vi "MC_10_19a.vi"() -> ()   [LabVIEW 2011]
uses:
  <vilib>/Utility/file.llb/Read From Spreadsheet File (string).vi
  <vilib>/Utility/inputDevices.llb/keyboardAcquire.vi
  <vilib>/Utility/file.llb/Write To Spreadsheet File (string).vi
  <vilib>/regexp/Match Regular Expression.xnode
panel:
  in  "Save Changes? 3":bool
  out "String":string
  in  "No Image":path=path "C:/Program Files/Mega Awesome/Image Not Found.png"
  in  "Save Changes? 2":bool
  in  "Project":path=path "C:/Program Files/Mega Awesome/DeviceData.opj"
  out "On/Off":dbl format="%#_3e"
  out "STS recorded":dbl
  out "Vt recorded":dbl
  out "Index 2":dbl
  out "Array 8":dbl[](array[numeric])
  out "Array 7":dbl[](array[numeric])
  in  "NumPts 2":dbl=5.0
  out "New S.T.S.":dbl
  out "S.T.S.":dbl
  in  "Slide 2":dbl(slide) step=1.0 scale=-1.0..82.0 scale format="%#_1p"
  in  "Previous Button 2":bool
  in  "Next Button 2":bool
  out "XY Graph 2":cluster{dbl[], dbl[]}[](graph)
  in  "Manual":bool
  out "New Vt":dbl
  out "Threshold V":dbl
  in  "Export":bool
  out "Image Name":string
  out "File":path
  out "Index":string
  out "Recorded Mobility":dbl format="%#_4e"
  in  "Remove Button":bool
  in  "Undo Button":bool
  out "Distances":dbl[](array[numeric])
  out "Total Width":dbl
  in  "Magnification":u16(ring) items=["5x", "10x", "20x", "50x", "80x"]
  out "Image Out":T1(plugin-control)
  in  "Folder":path
  out "Image Out 2":T1(plugin-control)
  out "ROI Descriptor out":T2 {"Contours"."Type" items=["No Selection", "Point", "Line", "Rectangle", "Oval", "Polygon", "Freehand Region", "Annulus", "Unused2", "Unused3", "Broken Line", "Freehand Line", "Rotated Rectangle"]}
  out "ROI Descriptor":T2 {"Contours"."Type" items=["No Selection", "Point", "Line", "Rectangle", "Oval", "Polygon", "Freehand Region", "Annulus", "Unused2", "Unused3", "Broken Line", "Freehand Line", "Rotated Rectangle"]}
  in  "Zoom":i16(slide)=-3 scale=-5.0..5.0
  out "Numeric 3":dbl
  in  "Blank Button":bool
  out "Array 6":dbl[][](array[numeric])
  out "Cluster":T3
  out "Array 5":dbl[](array[numeric])
  out "Array 4":dbl[](array[numeric])
  out "Array 3":dbl[](array[numeric])
  out "Numeric 2":dbl
  out "Numeric":dbl
  in  "Slide":dbl(slide) step=1.0 scale=-14.3..82.0 scale format="%#_1p"
  out "New Mobility":dbl format="%#_4e"
  out "Array 2":dbl[](array[numeric])
  out "Array":dbl[](array[numeric])
  in  "New Width":dbl
  in  "New Length":dbl
  in  "New Dielectric":dbl
  in  "Save Changes?":bool
  out "Index":dbl
  out "Data Name":string
  out "Folder":path
  in  "Down Button":bool
  in  "Up Button":bool
  in  "Previous Button":bool
  in  "Next Button":bool
  in  "Cancel Button":bool
  in  "NumPts":dbl=5.0
  out "XY Graph":cluster{dbl[], dbl[]}[](graph)
  out "Dielectric (d)":dbl
  out "Width":dbl
  out "Length":dbl
  out "Table Control 2":string[][](table)
  out "Table Control":string[][](table)
  in  "Row Start":dbl=20.0
  in  "File":path
  out "Mobility":dbl format="%#_4e"
  # "Data Location"
  # "Image Location"
  # "Recorded"
  # "Calculated"
  # "Re-Calculated"
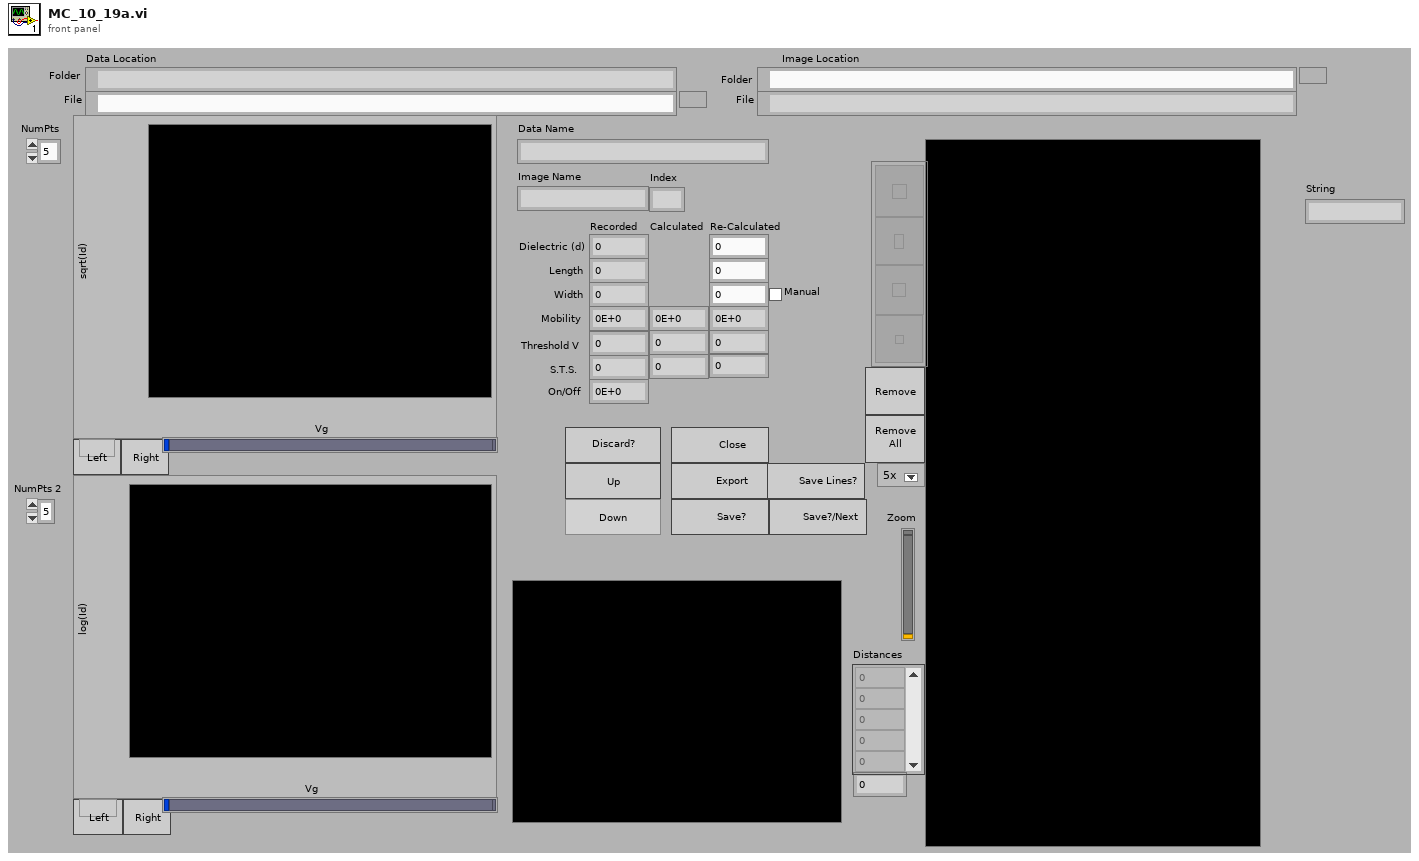
[diagram p1: front panel]
types:
  T1 = typedef "IMAQ Image.ctl" = refnum<image>
  T2 = typedef "ROI Descriptor" = cluster{"Global Rectangle":i32[], "Contours":cluster{"ID":enum32{"External", "Internal"}, "Type":u32, "Coordinates":i32[]}[]}
  T3 = cluster{"Numeric":dbl, "Numeric 2":dbl, "Numeric 3":dbl, "Numeric 4":dbl}
  T4 = cluster{"[0]":cluster{dbl[], dbl[]}, "[1]":cluster{dbl[], dbl[]}, "[2]":cluster{dbl[], dbl[]}, "[3]":cluster{dbl[], dbl[]}, "[4]":cluster{dbl[], dbl[]}, "[5]":cluster{dbl[], dbl[]}, "[6]":cluster{dbl[], dbl[]}, "[7]":cluster{dbl[], dbl[]}, "[8]":cluster{dbl[], dbl[]}}
  T5 = cluster{"Global Rectangle":i32[], "Contours":cluster{"Contour Type":u32, "ROI Type":u32, "Points":i32[]}[]}
  T6 = typedef "LVBoundsTypeDef.ctl" = cluster{"Width":u32, "Height":u32}
  T7 = cluster{"Contour Type":u32, "ROI Type":u32, "Points":i32[]}[]
  T8 = enum16{"0", "1", "2", "3", "4", "5", "6", "7", "8", "9", "A", "B", "C", "D", "E", "F", "G", "H", "I", "J", "K", "L", "M", "N", "O", "P", "Q", "R", "S", "T", "U", "V", "W", "X", "Y", "Z", "F1", "F2", "F3", "F4", "F5", "F6", "F7", "F8", "F9", "F10", "F11", "F12", "F13", "F14", "F15", "ADD", "BACK", "BACKSLASH", "CAPITAL", "COMMA", "DECIMAL", "DELETE", "DIVIDE", "DOWN", "END", "EQUALS", "ESCAPE", "GRAVE (`)", "HOME", "INSERT", "LBRACKET", "LCONTROL", "LEFT", "L ALT", "LSHIFT", "LWIN", "MINUS", "MULTIPLY", "NEXT", "NUMLOCK", "NUMPAD_0", "NUMPAD_1", "NUMPAD_2", "NUMPAD_3", "NUMPAD_4", "NUMPAD_5", "NUMPAD_6", "NUMPAD_7", "NUMPAD_8", "NUMPAD_9", "PAUSE", "PERIOD", "PRIOR (PG UP)", "RBRACKET", "RCONTROL", "RETURN", "RIGHT", "R ALT", "RSHIFT", "RWIN", "SCROLL", "SEMICOLON", "SLASH", "SPACE", "SUBTRACT", "TAB", "UP", "ENTER (num pad)", "' (quote)"}[]
  T9 = cluster{i32[], cluster{"Contour Type":u32, "ROI Type":u32, "Points":i32[]}[]}
  T10 = enum16{"0", "1", "2", "3", "4", "5", "6", "7", "8", "9", "A", "B", "C", "D", "E", "F", "G", "H", "I", "J", "K", "L", "M", "N", "O", "P", "Q", "R", "S", "T", "U", "V", "W", "X", "Y", "Z", "F1", "F2", "F3", "F4", "F5", "F6", "F7", "F8", "F9", "F10", "F11", "F12", "F13", "F14", "F15", "ADD", "BACK", "BACKSLASH", "CAPITAL", "COMMA", "DECIMAL", "DELETE", "DIVIDE", "DOWN", "END", "EQUALS", "ESCAPE", "GRAVE (`)", "HOME", "INSERT", "LBRACKET", "LCONTROL", "LEFT", "L ALT", "LSHIFT", "LWIN", "MINUS", "MULTIPLY", "NEXT", "NUMLOCK", "NUMPAD_0", "NUMPAD_1", "NUMPAD_2", "NUMPAD_3", "NUMPAD_4", "NUMPAD_5", "NUMPAD_6", "NUMPAD_7", "NUMPAD_8", "NUMPAD_9", "PAUSE", "PERIOD", "PRIOR (PG UP)", "RBRACKET", "RCONTROL", "RETURN", "RIGHT", "R ALT", "RSHIFT", "RWIN", "SCROLL", "SEMICOLON", "SLASH", "SPACE", "SUBTRACT", "TAB", "UP", "ENTER (num pad)", "' (quote)"}
  T11 = cluster{string, sgl, bool, bool, bool, bool, bool, bool, i32}
  T12 = cluster{i32, cluster{string, sgl, bool, bool, bool, bool, bool, bool, i32}, i32, i32}
  T13 = cluster{"Contour Type":u32, "ROI Type":u32, "Points":i32[]}
  T14 = cluster{"Points[0]":i32, "Points[1]":i32, "Points[2]":i32, "Points[3]":i32, "Points[4]":i32, "Points[5]":i32, "Points[6]":i32, "Points[7]":i32, "Points[8]":i32}
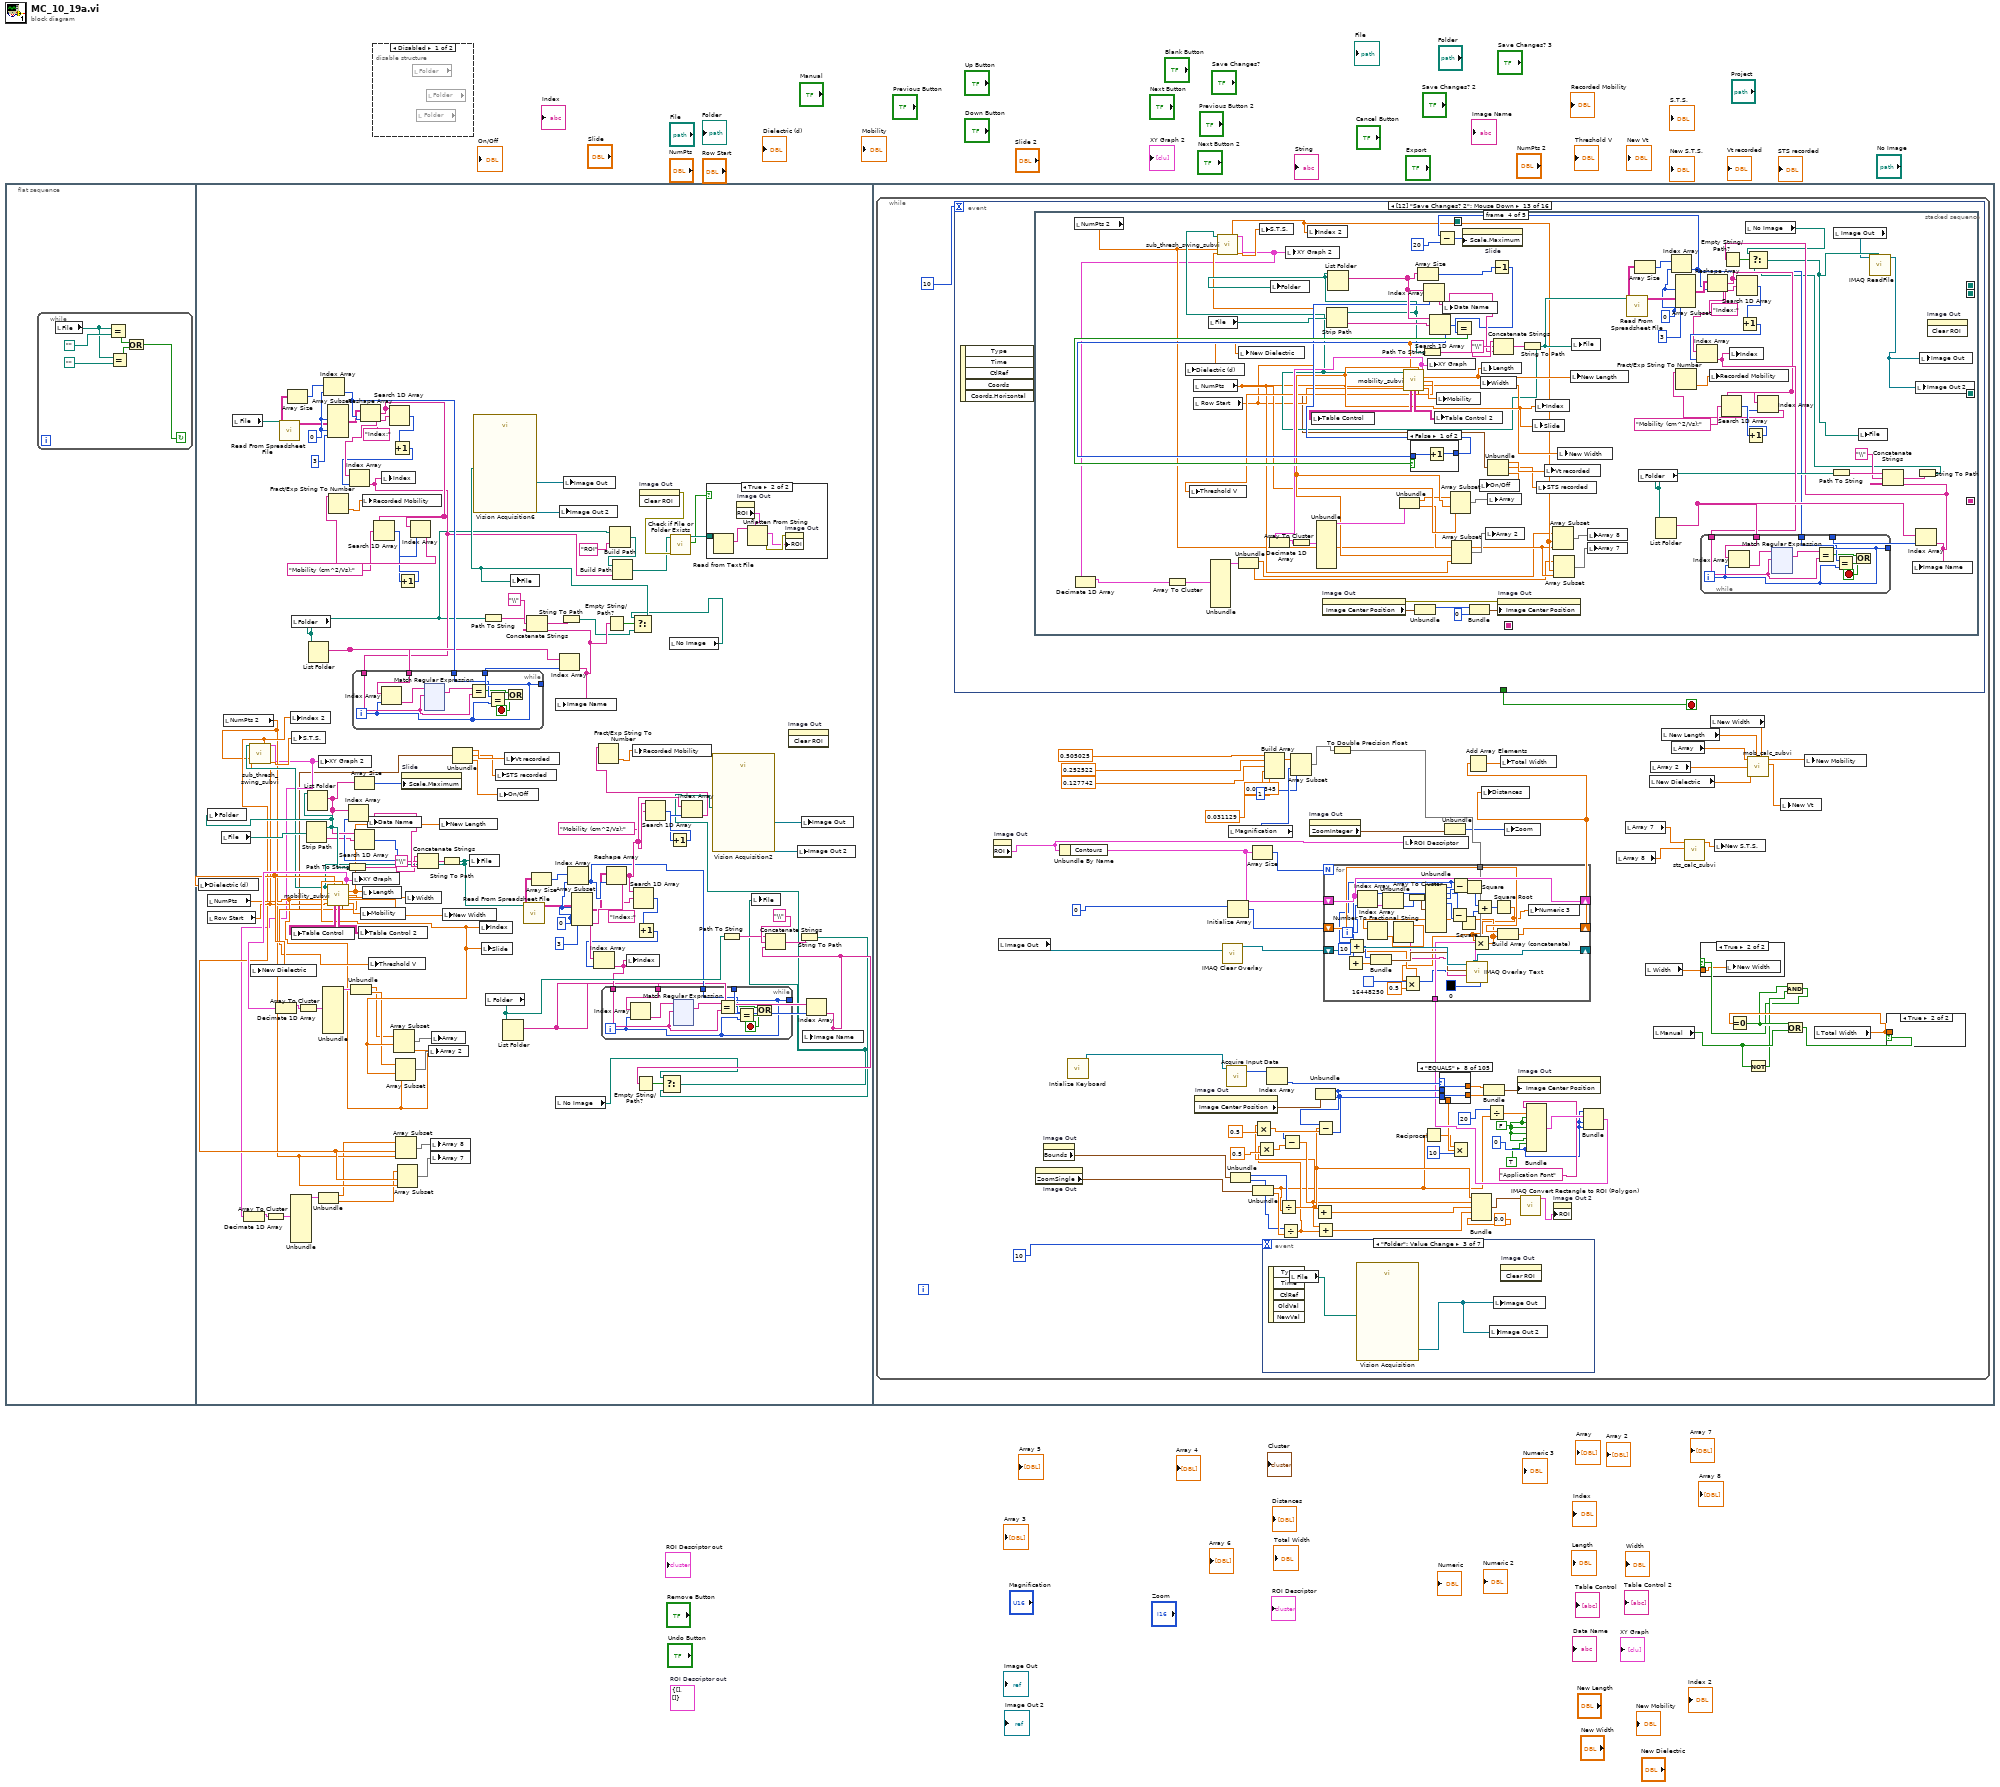
[diagram p0: block diagram]
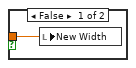
[diagram p4: hidden frame]
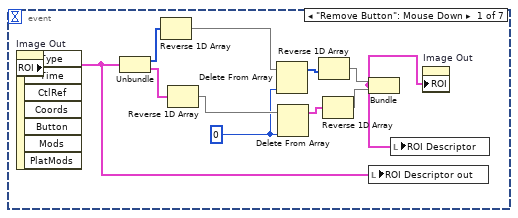
[diagram p5: hidden frame]
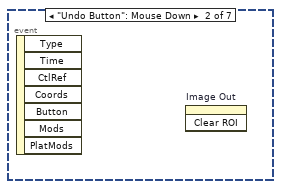
[diagram p6: hidden frame]
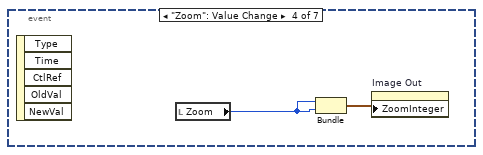
[diagram p7: hidden frame]
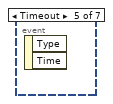
[diagram p8: hidden frame]
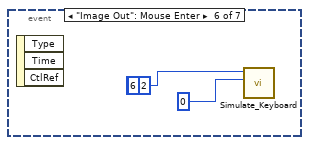
[diagram p9: hidden frame]
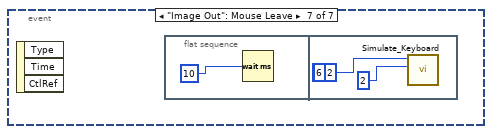
[diagram p10: hidden frame]
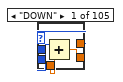
[diagram p11: hidden frame]
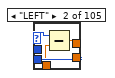
[diagram p12: hidden frame]
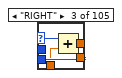
[diagram p13: hidden frame]
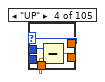
[diagram p14: hidden frame]
diagram:
  (unwired) T2 {"Global Rectangle"=[], "Contours"=[]}  # ROI Descriptor out
  n1 = flat-sequence {
    frame #0 {
      n2 = while {
        stop <- w1 continue-if-true
        n3 = local read "File"() -> (w3:path)
        n4 = Equal?(x=w3, y=path "") -> (x = y?=w5:bool)
        n5 = Equal?(x=w3, y=path "") -> (x = y?=w4:bool)
        n6 = Or(x=w5, y=w4) -> (x .or. y?=w1:bool)
      }
    }
    frame #1 {
      w67 = 0
      w97 = 0
      n7 = local read "NumPts"() -> (w42:dbl)
      n8 = local read "Row Start"() -> (w41:dbl)
      n9 = local read "File"() -> (w71:path)
      n10 = local read "NumPts 2"() -> (w36:dbl)
      n11 = local read "File"() -> (w92:path)
      n12 = call-poly <vilib>:"Read From Spreadsheet File.vi"("file path (dialog if empty)"=w92) -> ("all rows"=w95:string[][])  [unwired: 6 in, 4 out]
      n13 = Array Size(array=w95) -> (size(s)=w96:i32[])
      n14 = local read "Folder"() -> (w7:path)
      n15 = Strip Path(path=w71) -> (stripped path=w72:path, name=w53:string)
      n16 = local write "Folder"(w72) -> ()
      n17 = List Folder(path=w72) -> (filenames=w61:string[])  [unwired: 3 in, 3 out]
      n18 = List Folder(path=w7) -> (filenames=w101:string[])  [unwired: 3 in, 3 out]
      n19 = Index Array(array=w96, index=w97) -> (element=w103:i32)
      n20 = Array Subset(array=w95, index (row)=w97, index (col)=w97, length (col)=3) -> (w94:string[][])  [unwired: 1 in]
      n21 = Path To String(path=w72) -> (string=w52:string)
      n22 = Array Size(array=w61) -> (size(s)=w62:i32)
      n23 = Search 1D Array(1D array=w61, element=w53) -> (index of element=w60:i32)  [unwired: 1 in]
      n24 = Index Array(array=w61, index=w60) -> (element=w59:string)
      n25 = Reshape Array(w94, w103) -> (w113:string[])
      n26 = local write "Data Name"(w59) -> ()
      n27 = Search 1D Array(1D array=w113, element="Mobility (cm^2/Vs):") -> (index of element=w108:i32)  [unwired: 1 in]
      n28 = Search 1D Array(1D array=w113, element="Index:") -> (index of element=w100:i32)  [unwired: 1 in]
      n29 = Increment(x=w100) -> (x+1=w99:i32)
      n30 = Index Array(array=w113, index=w99) -> (element=w8:string)
      n31 = while {
        tunnel: w101 -> [w246]
        tunnel: w8 -> [w244]
        tunnel: [w243] -> _
        tunnel: [w243] -> w102
        tunnel: w103 -> [w242]
        i -> [w243]
        stop <- w239 stop-if-true
        n32 = Index Array(array=w246, index=w243) -> (element=w247:string)
        n33 = xnode "Match Regular Expression"("input string"=w247, "regular expression"=w244) -> ("whole match"=w245:string)  [unwired: 4 in, 4 out]
        n34 = Equal?(x=w245, y=w244) -> (x = y?=w241:bool)
        n35 = Equal?(x=w242, y=w243) -> (x = y?=w240:bool)
        n36 = Or(x=w241, y=w240) -> (x .or. y?=w239:bool)
      }
      n37 = local write "Index"(w8) -> ()
      n38 = Increment(x=w108) -> (x+1=w109:i32)
      n39 = property on="Slide" class="Slide (strict)"("Scale.Maximum"=w62) -> ()  [unwired: 2 in, 2 out]
      n40 = Index Array(array=w113, index=w109) -> (element=w111:string)
      n41 = Fract/Exp String To Number(string=w111) -> (number=w112:dbl)  [unwired: 3 in, 1 out]
      n42 = local write "Recorded Mobility"(w112) -> ()
      n43 = Concatenate Strings(w52, "\\", w59) -> (w54:string)
      n44 = String To Path(string=w54) -> (path=w43:path)
      n45 = call "sub_thresh_swing_subvi.vi"("Path"=w43, "NumPts"=w36, "Row Start"=w41) -> ("Index"=w37:dbl, "XY Graph"=w32:cluster{dbl[], dbl[]}[], "Sub Threshold Swing"=w44:dbl)  [unwired: 8 in, 2 out]
      n46 = Decimate 1D Array(w32) -> (w33:cluster{dbl[], dbl[]}[])  [unwired: 1 out]
      n47 = Array To Cluster(array=w33) -> (cluster=w35:T4)
      n48 = local write "Index 2"(w37) -> ()
      n49 = Unbundle(w35) -> ("[0]"=w34:cluster{dbl[], dbl[]})  [unwired: 8 out]
      n50 = local write "S.T.S."(w44) -> ()
      n51 = local write "XY Graph 2"(w32) -> ()
      n52 = Unbundle(w34) -> (w30:dbl[], w29:dbl[])
      n53 = call "mobility_subvi.vi"("Path"=w43, "NumPts"=w42, "Row Start"=w41) -> ("Dielectric (d)"=w48:dbl, "Index"=w49:dbl, "XY Graph"=w91:cluster{dbl[], dbl[]}[], "Length"=w47:dbl, "Vt"=w45:dbl, "Width"=w46:dbl, "Table Control"=w56:string[][], "Table Control 2"=w57:string[][], "Recorded"=w26:cluster{"Vt":dbl, "STS":dbl, "On/Off":dbl}, "Mobility"=w58:dbl)  [unwired: 3 in]
      n54 = local write "Dielectric (d)"(w48) -> ()
      n55 = local write "New Dielectric"(w48) -> ()
      n56 = Decimate 1D Array(w91) -> (w90:cluster{dbl[], dbl[]}[])  [unwired: 1 out]
      n57 = local write "Table Control"(w56) -> ()
      n58 = Array To Cluster(array=w90) -> (cluster=w88:T4)
      n59 = Unbundle(w88) -> ("[0]"=w89:cluster{dbl[], dbl[]})  [unwired: 8 out]
      n60 = Unbundle(w89) -> (w31:dbl[], w38:dbl[])
      n61 = local write "XY Graph"(w91) -> ()
      n62 = local write "Table Control 2"(w57) -> ()
      n63 = local write "Mobility"(w58) -> ()
      n64 = local write "Length"(w47) -> ()
      n65 = local write "Threshold V"(w45) -> ()
      n66 = Array Subset(array=w31, index=w49, length=w42) -> (w50:dbl[])
      n67 = Array Subset(array=w38, index=w49, length=w42) -> (w51:dbl[])
      n68 = Array Subset(array=w30, index=w37, length=w36) -> (w40:dbl[])
      n69 = Array Subset(array=w29, index=w37, length=w36) -> (w39:dbl[])
      n70 = local write "Width"(w46) -> ()
      n71 = local write "Array 2"(w51) -> ()
      n72 = local write "Array 8"(w40) -> ()
      n73 = local write "Array 7"(w39) -> ()
      n74 = local write "Array"(w50) -> ()
      n75 = local write "New Length"(w47) -> ()
      n76 = local write "New Width"(w46) -> ()
      n77 = Unbundle(w26) -> ("Vt"=w28:dbl, "STS"=w27:dbl, "On/Off"=w25:dbl)
      n78 = local write "File"(w43) -> ()
      n79 = local write "Index"(w49) -> ()
      n80 = local write "Slide"(w49) -> ()
      n81 = Path To String(path=w7) -> (string=w105:string)
      n82 = local read "Folder"() -> (w78:path)
      n83 = local write "STS recorded"(w27) -> ()
      n84 = local write "On/Off"(w25) -> ()
      n85 = List Folder(path=w78) -> (filenames=w74:string[])  [unwired: 3 in, 3 out]
      n86 = local write "Vt recorded"(w28) -> ()
      n87 = call-poly <vilib>:"Read From Spreadsheet File.vi"("file path (dialog if empty)"=w43) -> ("all rows"=w65:string[][])  [unwired: 6 in, 4 out]
      n88 = Array Size(array=w65) -> (size(s)=w66:i32[])
      n89 = local read "No Image"() -> (w16:path)
      n90 = Index Array(array=w101, index=w102) -> (element=w24:string)
      n91 = Concatenate Strings(w105, "\\", w24) -> (w106:string)
      n92 = local write "Image Name"(w24) -> ()
      n93 = String To Path(string=w106) -> (path=w22:path)
      n94 = Index Array(array=w66, index=w67) -> (element=w77:i32)
      n95 = Array Subset(array=w65, index (row)=w67, index (col)=w67, length (col)=3) -> (w64:string[][])  [unwired: 1 in]
      n96 = Empty String/Path?(string/path=w24) -> (empty?=w23:bool)
      n97 = Reshape Array(w64, w77) -> (w87:string[])
      n98 = Build Path(base path=w7, name or relative path="ROI") -> (appended path=w10:path)
      n99 = Build Path(base path=w10, name or relative path=w8) -> (appended path=w9:path)
      n100 = Search 1D Array(1D array=w87, element="Index:") -> (index of element=w70:i32)  [unwired: 1 in]
      n101 = Increment(x=w70) -> (x+1=w69:i32)
      n102 = Index Array(array=w87, index=w69) -> (element=w75:string)
      n103 = while {
        tunnel: w74 -> [w126]
        tunnel: w75 -> [w124]
        tunnel: [w123] -> _
        tunnel: [w123] -> w76
        tunnel: w77 -> [w122]
        i -> [w123]
        stop <- w119 stop-if-true
        n104 = Index Array(array=w126, index=w123) -> (element=w127:string)
        n105 = xnode "Match Regular Expression"("input string"=w127, "regular expression"=w124) -> ("whole match"=w125:string)  [unwired: 4 in, 4 out]
        n106 = Equal?(x=w125, y=w124) -> (x = y?=w121:bool)
        n107 = Equal?(x=w122, y=w123) -> (x = y?=w120:bool)
        n108 = Or(x=w121, y=w120) -> (x .or. y?=w119:bool)
      }
      n109 = local write "Index"(w75) -> ()
      n110 = invoke on="Image Out" class="ImageControl" method="Clear ROI"() -> (error out=w14:errorcluster)  [unwired: 3 in, 2 out]
      n111 = Search 1D Array(1D array=w87, element="Mobility (cm^2/Vs):") -> (index of element=w82:i32)  [unwired: 1 in]
      n112 = local read "No Image"() -> (w15:path)
      n113 = Select(t=w15, s=w23, f=w22) -> (s? t:f=w21:path)
      n114 = call "Vision Acquisition6"("Image Path"=w21) -> ("Image Out"=w104:T1)  [unwired: 25 in, 1 out]
      n115 = local write "File"(w21) -> ()
      n116 = local write "Image Out 2"(w104) -> ()
      n117 = local write "Image Out"(w104) -> ()
      n118 = Increment(x=w82) -> (x+1=w83:i32)
      n119 = call <vilib>:"Check if File or Folder Exists.vi"("error in (no error)"=w14, "path"=w9) -> ("file or folder exists?"=w12:bool, "dup path"=w13:path)  [unwired: 7 in, 1 out]
      n120 = Index Array(array=w87, index=w83) -> (element=w85:string)
      n121 = Fract/Exp String To Number(string=w85) -> (number=w86:dbl)  [unwired: 3 in, 1 out]
      n122 = local write "Recorded Mobility"(w86) -> ()
      n123 = case shown="True" w12 {
        tunnel: w13 -> [_ w114]
        frame False {
        }
        frame True {
          n124 = Read from Text File(file (use dialog)=w114) -> (text=w118:string)  [unwired: 3 in, 3 out]
          n125 = property on="Image Out" class="ImageControl"() -> ("ROI"=w115:T5)  [unwired: 2 in, 2 out]
          n126 = Unflatten From String(type=w115, binary string=w118) -> (value=w116:T5, error out=w117:errorcluster)  [unwired: 3 in, 1 out]
          n127 = property on="Image Out" class="ImageControl"(error in=w117, "ROI"=w116) -> ()  [unwired: 1 in, 2 out]
        }
      }
      n128 = Path To String(path=w78) -> (string=w79:string)
      n129 = invoke on="Image Out" class="ImageControl" method="Clear ROI"() -> ()  [unwired: 3 in, 3 out]
      n130 = Index Array(array=w74, index=w76) -> (element=w19:string)
      n131 = Empty String/Path?(string/path=w19) -> (empty?=w20:bool)
      n132 = Concatenate Strings(w79, "\\", w19) -> (w80:string)
      n133 = String To Path(string=w80) -> (path=w18:path)
      n134 = Select(t=w16, s=w20, f=w18) -> (s? t:f=w17:path)
      n135 = call "Vision Acquisition2"("Image Path"=w17) -> ("Image Out"=w73:T1)  [unwired: 25 in, 1 out]
      n136 = local write "File"(w17) -> ()
      n137 = local write "Image Out 2"(w73) -> ()
      n138 = local write "Image Out"(w73) -> ()
      n139 = local write "Image Name"(w19) -> ()
    }
    frame #2 {
      n140 = while {
        stop <- w438 stop-if-true
        w388 = FALSE
        w386 = 0
        n141 = event shown="[12] \"Save Changes? 2\": Mouse Down" {
          selector: _ -> [_ _ _ _ _ _ _ _ _ _ _ _ _ _ _ _]
          dyn-events: _ -> [_ _ _ _ _ _ _ _ _ _ _ _ _ _ _ _]
          timeout: 10 -> [_ _ _ _ _ _ _ _ _ _ _ _ _ _ _ _]
          tunnel: [_ _ _ _ _ _ _ _ _ _ _ _ _ TRUE _ TRUE] -> w438
          event Timeout {
            n142 = event-data() -> ()  [unwired: 1 in, 2 out]
          }
          event "Down Button": Mouse Down {
            w781 = 0
            n143 = event-data() -> ()  [unwired: 1 in, 7 out]
            n144 = local read "NumPts 2"() -> (w742:dbl)
            n145 = local read "NumPts"() -> (w749:dbl)
            n146 = local read "Row Start"() -> (w748:dbl)
            n147 = local read "File"() -> (w786:path)
            n148 = property on="Image Out" class="ImageControl"() -> (error out=w711:errorcluster, "Image Center Position"=w715:cluster{"X":u32, "Y":u32})  [unwired: 2 in, 1 out]
            n149 = Unbundle(w715) -> ("X"=w713:u32)  [unwired: 1 out]
            n150 = Strip Path(path=w786) -> (stripped path=w777:path, name=w799:string)
            n151 = local write "Folder"(w777) -> ()
            n152 = List Folder(path=w777) -> (filenames=w792:string[], error out=w720:errorcluster)  [unwired: 3 in, 2 out]
            n153 = Array Size(array=w792) -> (size(s)=w787:i32)
            n154 = Bundle("X"=w713, 0) -> (w714:cluster{"X":u32, i32})  [unwired: 1 in]
            n155 = Path To String(path=w777) -> (string=w800:string)
            n156 = Search 1D Array(1D array=w792, element=w799) -> (index of element=w789:i32)  [unwired: 1 in]
            n157 = property on="Image Out" class="ImageControl"(error in=w711, "Image Center Position"=w714) -> ()  [unwired: 1 in, 2 out]
            n158 = Decrement(x=w787) -> (x-1=w790:i32)
            n159 = Equal?(x=w789, y=w790) -> (x = y?=w791:bool)
            n160 = case shown="False" w791 {
              tunnel: w789 -> [w927 _]
              tunnel: [w926 0] -> w788
              frame False {
                n161 = Increment(x=w927) -> (x+1=w926:i32)
              }
              frame True {
              }
            }
            n162 = Index Array(array=w792, index=w788) -> (element=w793:string)
            n163 = local write "Data Name"(w793) -> ()
            n164 = Concatenate Strings(w800, "\\", w793) -> (w798:string)
            n165 = String To Path(string=w798) -> (path=w750:path)
            n166 = call "sub_thresh_swing_subvi.vi"("Path"=w750, "NumPts"=w742, "Row Start"=w748) -> ("Index"=w743:dbl, "XY Graph"=w738:cluster{dbl[], dbl[]}[], "Sub Threshold Swing"=w751:dbl)  [unwired: 8 in, 2 out]
            n167 = Decimate 1D Array(w738) -> (w741:cluster{dbl[], dbl[]}[])  [unwired: 1 out]
            n168 = Array To Cluster(array=w741) -> (cluster=w739:T4)
            n169 = Unbundle(w739) -> ("[0]"=w740:cluster{dbl[], dbl[]})  [unwired: 8 out]
            n170 = Unbundle(w740) -> (w737:dbl[], w736:dbl[])
            n171 = local write "S.T.S."(w751) -> ()
            n172 = local write "XY Graph 2"(w738) -> ()
            n173 = local write "Index 2"(w743) -> ()
            n174 = call "mobility_subvi.vi"("Path"=w750, "NumPts"=w749, "Row Start"=w748) -> ("Dielectric (d)"=w753:dbl, "Index"=w758:dbl, "XY Graph"=w761:cluster{dbl[], dbl[]}[], "Length"=w752:dbl, "Vt"=w754:dbl, "Width"=w726:dbl, "Table Control"=w796:string[][], "Table Control 2"=w795:string[][], "Recorded"=w735:cluster{"Vt":dbl, "STS":dbl, "On/Off":dbl}, "Mobility"=w794:dbl)  [unwired: 3 in]
            n175 = local write "Dielectric (d)"(w753) -> ()
            n176 = local write "Threshold V"(w754) -> ()
            n177 = local write "New Dielectric"(w753) -> ()
            n178 = Decimate 1D Array(w761) -> (w762:cluster{dbl[], dbl[]}[])  [unwired: 1 out]
            n179 = Array To Cluster(array=w762) -> (cluster=w764:T4)
            n180 = local write "Table Control"(w796) -> ()
            n181 = Unbundle(w764) -> ("[0]"=w763:cluster{dbl[], dbl[]})  [unwired: 8 out]
            n182 = Unbundle(w763) -> (w745:dbl[], w744:dbl[])
            n183 = local write "XY Graph"(w761) -> ()
            n184 = local write "Table Control 2"(w795) -> ()
            n185 = local write "Mobility"(w794) -> ()
            n186 = Array Subset(array=w745, index=w758, length=w749) -> (w760:dbl[])
            n187 = Array Subset(array=w744, index=w758, length=w749) -> (w759:dbl[])
            n188 = local write "Width"(w726) -> ()
            n189 = local write "Length"(w752) -> ()
            n190 = local write "Array 2"(w759) -> ()
            n191 = Unbundle(w735) -> ("Vt"=w734:dbl, "STS"=w733:dbl, "On/Off"=w732:dbl)
            n192 = local write "On/Off"(w732) -> ()
            n193 = local write "Array"(w760) -> ()
            n194 = local write "Slide"(w758) -> ()
            n195 = local write "Index"(w758) -> ()
            n196 = local write "STS recorded"(w733) -> ()
            n197 = local write "Vt recorded"(w734) -> ()
            n198 = Array Subset(array=w737, index=w743, length=w742) -> (w747:dbl[])
            n199 = Array Subset(array=w736, index=w743, length=w742) -> (w746:dbl[])
            n200 = local write "New Width"(w726) -> ()
            n201 = local write "New Length"(w752) -> ()
            n202 = local write "File"(w750) -> ()
            n203 = local write "Array 8"(w747) -> ()
            n204 = local write "Array 7"(w746) -> ()
            n205 = call-poly <vilib>:"Read From Spreadsheet File.vi"("file path (dialog if empty)"=w750) -> ("all rows"=w783:string[][])  [unwired: 6 in, 4 out]
            n206 = Array Size(array=w783) -> (size(s)=w782:i32[])
            n207 = local read "Folder"() -> (w717:path)
            n208 = List Folder(path=w717, error in=w720) -> (filenames=w776:string[], error out=w721:errorcluster)  [unwired: 2 in, 2 out]
            n209 = Index Array(array=w782, index=w781) -> (element=w756:i32)
            n210 = Subtract(x=w756, y=20) -> (x-y=w755:i32)
            n211 = property on="Slide" class="Slide (strict)"("Scale.Maximum"=w755) -> ()  [unwired: 2 in, 2 out]
            n212 = Array Subset(array=w783, index (row)=w781, index (col)=w781, length (col)=3) -> (w784:string[][])  [unwired: 1 in]
            n213 = Reshape Array(w784, w756) -> (w765:string[])
            n214 = local read "No Image"() -> (w727:path)
            n215 = Search 1D Array(1D array=w765, element="Mobility (cm^2/Vs):") -> (index of element=w770:i32)  [unwired: 1 in]
            n216 = Search 1D Array(1D array=w765, element="Index:") -> (index of element=w778:i32)  [unwired: 1 in]
            n217 = Increment(x=w778) -> (x+1=w779:i32)
            n218 = Index Array(array=w765, index=w779) -> (element=w719:string)
            n219 = while {
              tunnel: w776 -> [w813]
              tunnel: w719 -> [w811]
              tunnel: [w810] -> _
              tunnel: [w810] -> w775
              tunnel: w756 -> [w809]
              i -> [w810]
              stop <- w806 stop-if-true
              n220 = Index Array(array=w813, index=w810) -> (element=w814:string)
              n221 = xnode "Match Regular Expression"("input string"=w814, "regular expression"=w811) -> ("whole match"=w812:string)  [unwired: 4 in, 4 out]
              n222 = Equal?(x=w812, y=w811) -> (x = y?=w808:bool)
              n223 = Equal?(x=w809, y=w810) -> (x = y?=w807:bool)
              n224 = Or(x=w808, y=w807) -> (x .or. y?=w806:bool)
            }
            n225 = local write "Index"(w719) -> ()
            n226 = Increment(x=w770) -> (x+1=w769:i32)
            n227 = Build Path(base path=w717, name or relative path="ROI") -> (appended path=w716:path)
            n228 = Index Array(array=w765, index=w769) -> (element=w767:string)
            n229 = Fract/Exp String To Number(string=w767) -> (number=w766:dbl)  [unwired: 3 in, 1 out]
            n230 = local write "Recorded Mobility"(w766) -> ()
            n231 = Build Path(base path=w716, name or relative path=w719) -> (appended path=w725:path)
            n232 = Path To String(path=w717) -> (string=w773:string)
            n233 = invoke on="Image Out" class="ImageControl" method="Clear ROI"(error in=w721) -> (error out=w724:errorcluster)  [unwired: 2 in, 2 out]
            n234 = call <vilib>:"Check if File or Folder Exists.vi"("error in (no error)"=w724, "path"=w725) -> ("file or folder exists?"=w722:bool, "dup path"=w723:path)  [unwired: 7 in, 1 out]
            n235 = Index Array(array=w776, index=w775) -> (element=w730:string)
            n236 = Empty String/Path?(string/path=w730) -> (empty?=w731:bool)
            n237 = Concatenate Strings(w773, "\\", w730) -> (w772:string)
            n238 = local write "Image Name"(w730) -> ()
            n239 = String To Path(string=w772) -> (path=w729:path)
            n240 = Select(t=w727, s=w731, f=w729) -> (s? t:f=w728:path)
            n241 = call "Vision Acquisition4"("Image Path"=w728) -> ("Image Out"=w774:T1)  [unwired: 25 in, 1 out]
            n242 = local write "File"(w728) -> ()
            n243 = local write "Image Out 2"(w774) -> ()
            n244 = case shown="True" w722 {
              tunnel: w723 -> [_ w801]
              frame False {
              }
              frame True {
                n245 = Read from Text File(file (use dialog)=w801) -> (text=w805:string)  [unwired: 3 in, 3 out]
                n246 = property on="Image Out" class="ImageControl"() -> ("ROI"=w802:T5)  [unwired: 2 in, 2 out]
                n247 = Unflatten From String(type=w802, binary string=w805) -> (value=w803:T5, error out=w804:errorcluster)  [unwired: 3 in, 1 out]
                n248 = property on="Image Out" class="ImageControl"(error in=w804, "ROI"=w803) -> ()  [unwired: 1 in, 2 out]
              }
            }
            n249 = local write "Image Out"(w774) -> ()
            n250 = invoke on="Image Out" class="ImageControl" method="Clear ROI"() -> ()  [unwired: 3 in, 3 out]
          }
          event "File": Value Change {
            w1000 = 0
            n251 = event-data() -> ()  [unwired: 1 in, 5 out]
            n252 = local read "NumPts"() -> (w968:dbl)
            n253 = local read "Row Start"() -> (w967:dbl)
            n254 = local read "File"() -> (w996:path)
            n255 = local read "NumPts 2"() -> (w961:dbl)
            n256 = property on="Image Out" class="ImageControl"() -> (error out=w929:errorcluster, "Image Center Position"=w933:cluster{"X":u32, "Y":u32})  [unwired: 2 in, 1 out]
            n257 = Strip Path(path=w996) -> (stripped path=w995:path, name=w1013:string)
            n258 = local write "Folder"(w995) -> ()
            n259 = List Folder(path=w995) -> (filenames=w1005:string[], error out=w939:errorcluster)  [unwired: 3 in, 2 out]
            n260 = Unbundle(w933) -> ("X"=w931:u32)  [unwired: 1 out]
            n261 = Path To String(path=w995) -> (string=w1014:string)
            n262 = Search 1D Array(1D array=w1005, element=w1013) -> (index of element=w1006:i32)  [unwired: 1 in]
            n263 = Index Array(array=w1005, index=w1006) -> (element=w1007:string)
            n264 = Bundle("X"=w931, 0) -> (w932:cluster{"X":u32, i32})  [unwired: 1 in]
            n265 = local write "Data Name"(w1007) -> ()
            n266 = property on="Image Out" class="ImageControl"(error in=w929, "Image Center Position"=w932) -> ()  [unwired: 1 in, 2 out]
            n267 = Concatenate Strings(w1014, "\\", w1007) -> (w1012:string)
            n268 = String To Path(string=w1012) -> (path=w969:path)
            n269 = call "sub_thresh_swing_subvi.vi"("Path"=w969, "NumPts"=w961, "Row Start"=w967) -> ("Index"=w962:dbl, "XY Graph"=w957:cluster{dbl[], dbl[]}[], "Sub Threshold Swing"=w966:dbl)  [unwired: 8 in, 2 out]
            n270 = Decimate 1D Array(w957) -> (w960:cluster{dbl[], dbl[]}[])  [unwired: 1 out]
            n271 = Array To Cluster(array=w960) -> (cluster=w958:T4)
            n272 = Unbundle(w958) -> ("[0]"=w959:cluster{dbl[], dbl[]})  [unwired: 8 out]
            n273 = Unbundle(w959) -> (w955:dbl[], w954:dbl[])
            n274 = local write "Index 2"(w962) -> ()
            n275 = call "mobility_subvi.vi"("Path"=w969, "NumPts"=w968, "Row Start"=w967) -> ("Dielectric (d)"=w971:dbl, "Index"=w976:dbl, "XY Graph"=w979:cluster{dbl[], dbl[]}[], "Length"=w970:dbl, "Vt"=w972:dbl, "Width"=w944:dbl, "Table Control"=w1010:string[][], "Table Control 2"=w1009:string[][], "Recorded"=w951:cluster{"Vt":dbl, "STS":dbl, "On/Off":dbl}, "Mobility"=w1008:dbl)  [unwired: 3 in]
            n276 = local write "Dielectric (d)"(w971) -> ()
            n277 = local write "New Dielectric"(w971) -> ()
            n278 = Decimate 1D Array(w979) -> (w980:cluster{dbl[], dbl[]}[])  [unwired: 1 out]
            n279 = local write "Table Control"(w1010) -> ()
            n280 = Array To Cluster(array=w980) -> (cluster=w982:T4)
            n281 = Unbundle(w982) -> ("[0]"=w981:cluster{dbl[], dbl[]})  [unwired: 8 out]
            n282 = local write "Threshold V"(w972) -> ()
            n283 = local write "S.T.S."(w966) -> ()
            n284 = Unbundle(w981) -> (w956:dbl[], w963:dbl[])
            n285 = local write "XY Graph"(w979) -> ()
            n286 = local write "Table Control 2"(w1009) -> ()
            n287 = local write "Mobility"(w1008) -> ()
            n288 = local write "Length"(w970) -> ()
            n289 = local write "XY Graph 2"(w957) -> ()
            n290 = Unbundle(w951) -> ("Vt"=w953:dbl, "STS"=w952:dbl, "On/Off"=w950:dbl)
            n291 = local write "On/Off"(w950) -> ()
            n292 = Array Subset(array=w955, index=w962, length=w961) -> (w965:dbl[])
            n293 = Array Subset(array=w954, index=w962, length=w961) -> (w964:dbl[])
            n294 = local write "Width"(w944) -> ()
            n295 = Array Subset(array=w956, index=w976, length=w968) -> (w978:dbl[])
            n296 = Array Subset(array=w963, index=w976, length=w968) -> (w977:dbl[])
            n297 = local write "Array 8"(w965) -> ()
            n298 = local write "Array 7"(w964) -> ()
            n299 = local write "STS recorded"(w952) -> ()
            n300 = local write "Vt recorded"(w953) -> ()
            n301 = local write "New Length"(w970) -> ()
            n302 = local write "New Width"(w944) -> ()
            n303 = local write "Array 2"(w977) -> ()
            n304 = local write "Array"(w978) -> ()
            n305 = local write "File"(w969) -> ()
            n306 = local write "Index"(w976) -> ()
            n307 = local write "Slide"(w976) -> ()
            n308 = local read "Folder"() -> (w935:path)
            n309 = List Folder(path=w935, error in=w939) -> (filenames=w993:string[], error out=w938:errorcluster)  [unwired: 2 in, 2 out]
            n310 = call-poly <vilib>:"Read From Spreadsheet File.vi"("file path (dialog if empty)"=w969) -> ("all rows"=w1002:string[][])  [unwired: 6 in, 4 out]
            n311 = Array Size(array=w1002) -> (size(s)=w1001:i32[])
            n312 = Index Array(array=w1001, index=w1000) -> (element=w975:i32)
            n313 = Subtract(x=w975, y=20) -> (x-y=w973:i32)
            n314 = property on="Slide" class="Slide (strict)"("Scale.Maximum"=w973) -> ()  [unwired: 2 in, 2 out]
            n315 = Array Subset(array=w1002, index (row)=w1000, index (col)=w1000, length (col)=3) -> (w1003:string[][])  [unwired: 1 in]
            n316 = Reshape Array(w1003, w975) -> (w983:string[])
            n317 = Search 1D Array(1D array=w983, element="Index:") -> (index of element=w997:i32)  [unwired: 1 in]
            n318 = Increment(x=w997) -> (x+1=w998:i32)
            n319 = Index Array(array=w983, index=w998) -> (element=w937:string)
            n320 = while {
              tunnel: w993 -> [w1027]
              tunnel: w937 -> [w1025]
              tunnel: [w1024] -> _
              tunnel: [w1024] -> w992
              tunnel: w975 -> [w1023]
              i -> [w1024]
              stop <- w1020 stop-if-true
              n321 = Index Array(array=w1027, index=w1024) -> (element=w1028:string)
              n322 = xnode "Match Regular Expression"("input string"=w1028, "regular expression"=w1025) -> ("whole match"=w1026:string)  [unwired: 4 in, 4 out]
              n323 = Equal?(x=w1026, y=w1025) -> (x = y?=w1022:bool)
              n324 = Equal?(x=w1023, y=w1024) -> (x = y?=w1021:bool)
              n325 = Or(x=w1022, y=w1021) -> (x .or. y?=w1020:bool)
            }
            n326 = local write "Index"(w937) -> ()
            n327 = Search 1D Array(1D array=w983, element="Mobility (cm^2/Vs):") -> (index of element=w988:i32)  [unwired: 1 in]
            n328 = Increment(x=w988) -> (x+1=w987:i32)
            n329 = Index Array(array=w983, index=w987) -> (element=w985:string)
            n330 = Fract/Exp String To Number(string=w985) -> (number=w984:dbl)  [unwired: 3 in, 1 out]
            n331 = local write "Recorded Mobility"(w984) -> ()
            n332 = Build Path(base path=w935, name or relative path="ROI") -> (appended path=w934:path)
            n333 = Path To String(path=w935) -> (string=w991:string)
            n334 = local read "No Image"() -> (w945:path)
            n335 = Build Path(base path=w934, name or relative path=w937) -> (appended path=w943:path)
            n336 = invoke on="Image Out" class="ImageControl" method="Clear ROI"(error in=w938) -> (error out=w942:errorcluster)  [unwired: 2 in, 2 out]
            n337 = Index Array(array=w993, index=w992) -> (element=w948:string)
            n338 = Empty String/Path?(string/path=w948) -> (empty?=w949:bool)
            n339 = Concatenate Strings(w991, "\\", w948) -> (w990:string)
            n340 = String To Path(string=w990) -> (path=w947:path)
            n341 = Select(t=w945, s=w949, f=w947) -> (s? t:f=w946:path)
            n342 = call "Vision Acquisition3"("Image Path"=w946) -> ("Image Out"=w994:T1)  [unwired: 25 in, 1 out]
            n343 = local write "File"(w946) -> ()
            n344 = local write "Image Out 2"(w994) -> ()
            n345 = local write "Image Out"(w994) -> ()
            n346 = local write "Image Name"(w948) -> ()
            n347 = call <vilib>:"Check if File or Folder Exists.vi"("error in (no error)"=w942, "path"=w943) -> ("file or folder exists?"=w940:bool, "dup path"=w941:path)  [unwired: 7 in, 1 out]
            n348 = invoke on="Image Out" class="ImageControl" method="Clear ROI"() -> ()  [unwired: 3 in, 3 out]
            n349 = case shown="True" w940 {
              tunnel: w941 -> [_ w1015]
              frame False {
              }
              frame True {
                n350 = Read from Text File(file (use dialog)=w1015) -> (text=w1019:string)  [unwired: 3 in, 3 out]
                n351 = property on="Image Out" class="ImageControl"() -> ("ROI"=w1016:T5)  [unwired: 2 in, 2 out]
                n352 = Unflatten From String(type=w1016, binary string=w1019) -> (value=w1017:T5, error out=w1018:errorcluster)  [unwired: 3 in, 1 out]
                n353 = property on="Image Out" class="ImageControl"(error in=w1018, "ROI"=w1017) -> ()  [unwired: 1 in, 2 out]
              }
            }
          }
          event "Up Button": Mouse Down {
            w1211 = 0
            n354 = event-data() -> ()  [unwired: 1 in, 5 out]
            n355 = local read "NumPts"() -> (w1182:dbl)
            n356 = local read "Row Start"() -> (w1181:dbl)
            n357 = local read "NumPts 2"() -> (w1176:dbl)
            n358 = local read "File"() -> (w1207:path)
            n359 = property on="Image Out" class="ImageControl"() -> (error out=w1140:errorcluster, "Image Center Position"=w1144:cluster{"X":u32, "Y":u32})  [unwired: 2 in, 1 out]
            n360 = Strip Path(path=w1207) -> (stripped path=w1206:path, name=w1227:string)
            n361 = local write "Folder"(w1206) -> ()
            n362 = List Folder(path=w1206) -> (filenames=w1217:string[], error out=w1150:errorcluster)  [unwired: 3 in, 2 out]
            n363 = Path To String(path=w1206) -> (string=w1228:string)
            n364 = Search 1D Array(1D array=w1217, element=w1227) -> (index of element=w1219:i32)  [unwired: 1 in]
            n365 = Equal To 0?(x=w1219) -> (x = 0?=w1220:bool)
            n366 = Unbundle(w1144) -> ("X"=w1142:u32)  [unwired: 1 out]
            n367 = Bundle("X"=w1142, 0) -> (w1143:cluster{"X":u32, i32})  [unwired: 1 in]
            n368 = property on="Image Out" class="ImageControl"(error in=w1140, "Image Center Position"=w1143) -> ()  [unwired: 1 in, 2 out]
            n369 = Array Size(array=w1217) -> (size(s)=w1216:i32)
            n370 = case shown="True" w1220 {
              tunnel: w1219 -> [w1355 _]
              tunnel: [w1354 w1356] -> w1218
              tunnel: w1216 -> [_ w1357]
              frame False {
                n371 = Decrement(x=w1355) -> (x-1=w1354:i32)
              }
              frame True {
                n372 = Decrement(x=w1357) -> (x-1=w1356:i32)
              }
            }
            n373 = Index Array(array=w1217, index=w1218) -> (element=w1221:string)
            n374 = local write "Data Name"(w1221) -> ()
            n375 = Concatenate Strings(w1228, "\\", w1221) -> (w1226:string)
            n376 = String To Path(string=w1226) -> (path=w1183:path)
            n377 = call "sub_thresh_swing_subvi.vi"("Path"=w1183, "NumPts"=w1176, "Row Start"=w1181) -> ("Index"=w1175:dbl, "XY Graph"=w1171:cluster{dbl[], dbl[]}[], "Sub Threshold Swing"=w1184:dbl)  [unwired: 8 in, 2 out]
            n378 = Decimate 1D Array(w1171) -> (w1174:cluster{dbl[], dbl[]}[])  [unwired: 1 out]
            n379 = Array To Cluster(array=w1174) -> (cluster=w1172:T4)
            n380 = Unbundle(w1172) -> ("[0]"=w1173:cluster{dbl[], dbl[]})  [unwired: 8 out]
            n381 = Unbundle(w1173) -> (w1170:dbl[], w1169:dbl[])
            n382 = Array Subset(array=w1170, index=w1175, length=w1176) -> (w1178:dbl[])
            n383 = Array Subset(array=w1169, index=w1175, length=w1176) -> (w1177:dbl[])
            n384 = local write "S.T.S."(w1184) -> ()
            n385 = local write "Array 8"(w1178) -> ()
            n386 = local write "Array 7"(w1177) -> ()
            n387 = call "mobility_subvi.vi"("Path"=w1183, "NumPts"=w1182, "Row Start"=w1181) -> ("Dielectric (d)"=w1186:dbl, "Index"=w1188:dbl, "XY Graph"=w1194:cluster{dbl[], dbl[]}[], "Length"=w1185:dbl, "Vt"=w1187:dbl, "Width"=w1162:dbl, "Table Control"=w1224:string[][], "Table Control 2"=w1223:string[][], "Recorded"=w1166:cluster{"Vt":dbl, "STS":dbl, "On/Off":dbl}, "Mobility"=w1222:dbl)  [unwired: 3 in]
            n388 = local write "Dielectric (d)"(w1186) -> ()
            n389 = local write "New Dielectric"(w1186) -> ()
            n390 = local write "New Length"(w1185) -> ()
            n391 = local write "New Width"(w1162) -> ()
            n392 = local write "Table Control"(w1224) -> ()
            n393 = Decimate 1D Array(w1194) -> (w1195:cluster{dbl[], dbl[]}[])  [unwired: 1 out]
            n394 = local write "XY Graph 2"(w1171) -> ()
            n395 = Array To Cluster(array=w1195) -> (cluster=w1197:T4)
            n396 = local write "XY Graph"(w1194) -> ()
            n397 = local write "Index 2"(w1175) -> ()
            n398 = local write "Table Control 2"(w1223) -> ()
            n399 = local write "Mobility"(w1222) -> ()
            n400 = local write "Length"(w1185) -> ()
            n401 = Unbundle(w1197) -> ("[0]"=w1196:cluster{dbl[], dbl[]})  [unwired: 8 out]
            n402 = Unbundle(w1196) -> (w1180:dbl[], w1179:dbl[])
            n403 = local write "Threshold V"(w1187) -> ()
            n404 = local write "Width"(w1162) -> ()
            n405 = Unbundle(w1166) -> ("Vt"=w1168:dbl, "STS"=w1167:dbl, "On/Off"=w1165:dbl)
            n406 = Array Subset(array=w1180, index=w1188, length=w1182) -> (w1193:dbl[])
            n407 = Array Subset(array=w1179, index=w1188, length=w1182) -> (w1192:dbl[])
            n408 = local write "STS recorded"(w1167) -> ()
            n409 = local write "Index"(w1188) -> ()
            n410 = local write "Vt recorded"(w1168) -> ()
            n411 = local write "File"(w1183) -> ()
            n412 = local write "On/Off"(w1165) -> ()
            n413 = local write "Array 2"(w1192) -> ()
            n414 = local write "Array"(w1193) -> ()
            n415 = local read "Folder"() -> (w1154:path)
            n416 = local write "Slide"(w1188) -> ()
            n417 = List Folder(path=w1154, error in=w1150) -> (filenames=w1205:string[], error out=w1149:errorcluster)  [unwired: 2 in, 2 out]
            n418 = call-poly <vilib>:"Read From Spreadsheet File.vi"("file path (dialog if empty)"=w1183) -> ("all rows"=w1213:string[][])  [unwired: 6 in, 4 out]
            n419 = Array Size(array=w1213) -> (size(s)=w1212:i32[])
            n420 = Index Array(array=w1212, index=w1211) -> (element=w1190:i32)
            n421 = Subtract(x=w1190, y=20) -> (x-y=w1189:i32)
            n422 = property on="Slide" class="Slide (strict)"("Scale.Maximum"=w1189) -> ()  [unwired: 2 in, 2 out]
            n423 = Array Subset(array=w1213, index (row)=w1211, index (col)=w1211, length (col)=3) -> (w1214:string[][])  [unwired: 1 in]
            n424 = Reshape Array(w1214, w1190) -> (w1200:string[])
            n425 = Search 1D Array(1D array=w1200, element="Mobility (cm^2/Vs):") -> (index of element=w1203:i32)  [unwired: 1 in]
            n426 = Increment(x=w1203) -> (x+1=w1202:i32)
            n427 = Index Array(array=w1200, index=w1202) -> (element=w1199:string)
            n428 = Fract/Exp String To Number(string=w1199) -> (number=w1198:dbl)  [unwired: 3 in, 1 out]
            n429 = local write "Recorded Mobility"(w1198) -> ()
            n430 = Search 1D Array(1D array=w1200, element="Index:") -> (index of element=w1208:i32)  [unwired: 1 in]
            n431 = Increment(x=w1208) -> (x+1=w1209:i32)
            n432 = Index Array(array=w1200, index=w1209) -> (element=w1146:string)
            n433 = while {
              tunnel: w1205 -> [w1241]
              tunnel: w1146 -> [w1239]
              tunnel: [w1238] -> w1204
              tunnel: w1190 -> [w1237]
              i -> [w1238]
              stop <- w1234 stop-if-true
              n434 = Index Array(array=w1241, index=w1238) -> (element=w1242:string)
              n435 = xnode "Match Regular Expression"("input string"=w1242, "regular expression"=w1239) -> ("whole match"=w1240:string)  [unwired: 4 in, 4 out]
              n436 = Equal?(x=w1240, y=w1239) -> (x = y?=w1236:bool)
              n437 = Equal?(x=w1237, y=w1238) -> (x = y?=w1235:bool)
              n438 = Or(x=w1236, y=w1235) -> (x .or. y?=w1234:bool)
            }
            n439 = local write "Index"(w1146) -> ()
            n440 = Build Path(base path=w1154, name or relative path="ROI") -> (appended path=w1147:path)
            n441 = Build Path(base path=w1147, name or relative path=w1146) -> (appended path=w1145:path)
            n442 = invoke on="Image Out" class="ImageControl" method="Clear ROI"(error in=w1149) -> (error out=w1153:errorcluster)  [unwired: 2 in, 2 out]
            n443 = call <vilib>:"Check if File or Folder Exists.vi"("error in (no error)"=w1153, "path"=w1145) -> ("file or folder exists?"=w1151:bool, "dup path"=w1152:path)  [unwired: 7 in, 1 out]
            n444 = local read "No Image"() -> (w1163:path)
            n445 = Index Array(array=w1205, index=w1204) -> (element=w1156:string)
            n446 = Build Path(base path=w1154, name or relative path=w1156) -> (appended path=w1155:path)
            n447 = local write "Image Name"(w1156) -> ()
            n448 = case shown="True" w1151 {
              tunnel: w1152 -> [_ w1229]
              frame False {
              }
              frame True {
                n449 = Read from Text File(file (use dialog)=w1229) -> (text=w1233:string)  [unwired: 3 in, 3 out]
                n450 = property on="Image Out" class="ImageControl"() -> ("ROI"=w1230:T5)  [unwired: 2 in, 2 out]
                n451 = Unflatten From String(type=w1230, binary string=w1233) -> (value=w1231:T5, error out=w1232:errorcluster)  [unwired: 3 in, 1 out]
                n452 = property on="Image Out" class="ImageControl"(error in=w1232, "ROI"=w1231) -> ()  [unwired: 1 in, 2 out]
              }
            }
            n453 = Empty String/Path?(string/path=w1156) -> (empty?=w1164:bool)
            n454 = Select(t=w1163, s=w1164, f=w1155) -> (s? t:f=w1157:path)
            n455 = call "Vision Acquisition5"("Image Path"=w1157) -> ("Image Out"=w1161:T1)  [unwired: 25 in, 1 out]
            n456 = local write "File"(w1157) -> ()
            n457 = local write "Image Out 2"(w1161) -> ()
            n458 = local write "Image Out"(w1161) -> ()
            n459 = call <vilib>:"Get File Extension.vi"("file"=w1157) -> ("lowercase file extension"=w1159:string)  [unwired: 7 in, 3 out]
            n460 = local write "String"(w1159) -> ()
            n461 = Search 1D Array(1D array=string[] ["bmp", "jpeg", "png", "jpg", "gif"], element=w1159) -> (index of element=w1158:i32)  [unwired: 1 in]
            n462 = Less Than 0?(x=w1158) -> ()  [unwired: 1 out]
          }
          event "Save Changes? 3": Mouse Down {
            n463 = event-data() -> ()  [unwired: 1 in, 7 out]
            n464 = local read "Folder"() -> (w1358:path)
            n465 = Build Path(base path=w1358, name or relative path="ROI") -> (appended path=w1365:path)
            n466 = call <vilib>:"Check if File or Folder Exists.vi"("path"=w1365) -> ("file or folder exists?"=w1367:bool, "dup path"=w1364:path)  [unwired: 8 in, 1 out]
            n467 = case shown="False" w1367 {
              tunnel: w1364 -> [w1369 w1370]
              tunnel: [w1368 w1370] -> w1359
              frame False {
                n468 = Create Folder(path (use dialog)=w1369) -> (created path=w1368:path)  [unwired: 2 in, 2 out]
              }
              frame True {
              }
            }
            n469 = property on="Image Out" class="ImageControl"() -> ("ROI"=w1363:T5)  [unwired: 2 in, 2 out]
            n470 = local read "Index"() -> (w1361:string)
            n471 = Flatten To String(anything=w1363) -> (data string=w1362:string)  [unwired: 3 in, 2 out]
            n472 = Build Path(base path=w1359, name or relative path=w1361) -> (appended path=w1360:path)
            n473 = Write to Text File(file (use dialog)=w1360, text=w1362) -> ()  [unwired: 2 in, 3 out]
          }
          event "Next Button": Mouse Down {
            n474 = event-data() -> ()  [unwired: 1 in, 5 out]
            n475 = local read "XY Graph"() -> (w1383:cluster{dbl[], dbl[]}[])
            n476 = local read "NumPts"() -> (w1384:dbl)
            n477 = local read "Index"() -> (w1385:dbl)
            n478 = Decimate 1D Array(w1383) -> (w1379:cluster{dbl[], dbl[]}[], w1378:cluster{dbl[], dbl[]}[])
            n479 = Array To Cluster(array=w1379) -> (cluster=w1389:T4)
            n480 = Unbundle(w1389) -> ("[0]"=w1388:cluster{dbl[], dbl[]})  [unwired: 8 out]
            n481 = Increment(x=w1385) -> (x+1=w1380:dbl)
            n482 = Unbundle(w1388) -> (w1387:dbl[], w1386:dbl[])
            n483 = Array Subset(array=w1387, index=w1380, length=w1384) -> (w1376:dbl[])
            n484 = local write "Index"(w1380) -> ()
            n485 = Array Subset(array=w1386, index=w1380, length=w1384) -> (w1375:dbl[])
            n486 = Bundle(w1376, w1375) -> (w1382:cluster{dbl[], dbl[]})  [unwired: 1 in]
            n487 = Build Array (concatenate)(w1379, w1378, w1382) -> (w1381:cluster{dbl[], dbl[]}[])
            n488 = local write "XY Graph"(w1381) -> ()
            n489 = local read "New Dielectric"() -> (w1374:dbl)
            n490 = local write "Array 2"(w1375) -> ()
            n491 = local read "New Length"() -> (w1373:dbl)
            n492 = local write "Array"(w1376) -> ()
            n493 = local read "New Width"() -> (w1372:dbl)
            n494 = call "mob_calc_subvi.vi"("Width"=w1372, "Length"=w1373, "Dielectric (d)"=w1374, "Array 2"=w1375, "Array"=w1376) -> ("Vt"=w1371:dbl, "Mobility"=w1377:dbl)  [unwired: 5 in]
            n495 = local write "New Mobility"(w1377) -> ()
            n496 = local write "New Vt"(w1371) -> ()
          }
          event "Next Button 2": Mouse Down {
            n497 = event-data() -> ()  [unwired: 1 in, 7 out]
            n498 = local read "XY Graph 2"() -> (w1398:cluster{dbl[], dbl[]}[])
            n499 = local read "Index 2"() -> (w1400:dbl)
            n500 = local read "NumPts 2"() -> (w1399:dbl)
            n501 = Decimate 1D Array(w1398) -> (w1394:cluster{dbl[], dbl[]}[], w1393:cluster{dbl[], dbl[]}[])
            n502 = Array To Cluster(array=w1394) -> (cluster=w1404:T4)
            n503 = Unbundle(w1404) -> ("[0]"=w1403:cluster{dbl[], dbl[]})  [unwired: 8 out]
            n504 = Increment(x=w1400) -> (x+1=w1395:dbl)
            n505 = Unbundle(w1403) -> (w1402:dbl[], w1401:dbl[])
            n506 = local write "Index 2"(w1395) -> ()
            n507 = Array Subset(array=w1402, index=w1395, length=w1399) -> (w1391:dbl[])
            n508 = Array Subset(array=w1401, index=w1395, length=w1399) -> (w1390:dbl[])
            n509 = Bundle(w1391, w1390) -> (w1397:cluster{dbl[], dbl[]})  [unwired: 1 in]
            n510 = Build Array (concatenate)(w1394, w1393, w1397) -> (w1396:cluster{dbl[], dbl[]}[])
            n511 = local write "XY Graph 2"(w1396) -> ()
            n512 = local write "Array 8"(w1391) -> ()
            n513 = call "sts_calc_subvi.vi"("Array 2"=w1391, "Array"=w1390) -> ("STS"=w1392:dbl)  [unwired: 9 in]
            n514 = local write "Array 7"(w1390) -> ()
            n515 = local write "New S.T.S."(w1392) -> ()
          }
          event "Previous Button 2": Mouse Down {
            n516 = event-data() -> ()  [unwired: 1 in, 7 out]
            n517 = local read "XY Graph 2"() -> (w1414:cluster{dbl[], dbl[]}[])
            n518 = local read "NumPts 2"() -> (w1415:dbl)
            n519 = local read "Index 2"() -> (w1407:dbl)
            n520 = Decimate 1D Array(w1414) -> (w1411:cluster{dbl[], dbl[]}[], w1410:cluster{dbl[], dbl[]}[])
            n521 = Array To Cluster(array=w1411) -> (cluster=w1419:T4)
            n522 = Unbundle(w1419) -> ("[0]"=w1418:cluster{dbl[], dbl[]})  [unwired: 8 out]
            n523 = Decrement(x=w1407) -> (x-1=w1408:dbl)
            n524 = Unbundle(w1418) -> (w1417:dbl[], w1416:dbl[])
            n525 = local write "Index 2"(w1408) -> ()
            n526 = Array Subset(array=w1417, index=w1408, length=w1415) -> (w1405:dbl[])
            n527 = Array Subset(array=w1416, index=w1408, length=w1415) -> (w1406:dbl[])
            n528 = Bundle(w1405, w1406) -> (w1413:cluster{dbl[], dbl[]})  [unwired: 1 in]
            n529 = Build Array (concatenate)(w1411, w1410, w1413) -> (w1412:cluster{dbl[], dbl[]}[])
            n530 = local write "XY Graph 2"(w1412) -> ()
            n531 = local write "Array 7"(w1406) -> ()
            n532 = call "sts_calc_subvi.vi"("Array 2"=w1405, "Array"=w1406) -> ("STS"=w1409:dbl)  [unwired: 9 in]
            n533 = local write "Array 8"(w1405) -> ()
            n534 = local write "New S.T.S."(w1409) -> ()
          }
          event "Previous Button": Mouse Down {
            n535 = event-data() -> ()  [unwired: 1 in, 5 out]
            n536 = local read "XY Graph"() -> (w1433:cluster{dbl[], dbl[]}[])
            n537 = Decimate 1D Array(w1433) -> (w1430:cluster{dbl[], dbl[]}[], w1429:cluster{dbl[], dbl[]}[])
            n538 = local read "NumPts"() -> (w1434:dbl)
            n539 = local read "Index"() -> (w1428:dbl)
            n540 = Array To Cluster(array=w1430) -> (cluster=w1438:T4)
            n541 = Unbundle(w1438) -> ("[0]"=w1437:cluster{dbl[], dbl[]})  [unwired: 8 out]
            n542 = Decrement(x=w1428) -> (x-1=w1427:dbl)
            n543 = Unbundle(w1437) -> (w1436:dbl[], w1435:dbl[])
            n544 = local read "New Dielectric"() -> (w1421:dbl)
            n545 = Array Subset(array=w1436, index=w1427, length=w1434) -> (w1426:dbl[])
            n546 = Array Subset(array=w1435, index=w1427, length=w1434) -> (w1425:dbl[])
            n547 = local write "Index"(w1427) -> ()
            n548 = Bundle(w1426, w1425) -> (w1432:cluster{dbl[], dbl[]})  [unwired: 1 in]
            n549 = Build Array (concatenate)(w1430, w1429, w1432) -> (w1431:cluster{dbl[], dbl[]}[])
            n550 = local write "XY Graph"(w1431) -> ()
            n551 = local read "New Length"() -> (w1422:dbl)
            n552 = local write "Array 2"(w1425) -> ()
            n553 = local read "New Width"() -> (w1423:dbl)
            n554 = call "mob_calc_subvi.vi"("Width"=w1423, "Length"=w1422, "Dielectric (d)"=w1421, "Array 2"=w1425, "Array"=w1426) -> ("Vt"=w1420:dbl, "Mobility"=w1424:dbl)  [unwired: 5 in]
            n555 = local write "New Mobility"(w1424) -> ()
            n556 = local write "Array"(w1426) -> ()
            n557 = local write "New Vt"(w1420) -> ()
          }
          event "Slide": Value Change {
            n558 = event-data() -> ()  [unwired: 1 in, 5 out]
            n559 = local read "XY Graph"() -> (w1451:cluster{dbl[], dbl[]}[])
            n560 = local read "Slide"() -> (w1440:dbl)
            n561 = Decimate 1D Array(w1451) -> (w1448:cluster{dbl[], dbl[]}[], w1447:cluster{dbl[], dbl[]}[])
            n562 = local read "NumPts"() -> (w1452:dbl)
            n563 = Array To Cluster(array=w1448) -> (cluster=w1456:T4)
            n564 = Unbundle(w1456) -> ("[0]"=w1455:cluster{dbl[], dbl[]})  [unwired: 8 out]
            n565 = Unbundle(w1455) -> (w1454:dbl[], w1453:dbl[])
            n566 = local read "New Dielectric"() -> (w1441:dbl)
            n567 = Array Subset(array=w1454, index=w1440, length=w1452) -> (w1446:dbl[])
            n568 = Array Subset(array=w1453, index=w1440, length=w1452) -> (w1445:dbl[])
            n569 = local write "Index"(w1440) -> ()
            n570 = Bundle(w1446, w1445) -> (w1450:cluster{dbl[], dbl[]})  [unwired: 1 in]
            n571 = Build Array (concatenate)(w1448, w1447, w1450) -> (w1449:cluster{dbl[], dbl[]}[])
            n572 = local write "XY Graph"(w1449) -> ()
            n573 = local read "New Length"() -> (w1442:dbl)
            n574 = local write "Array 2"(w1445) -> ()
            n575 = local read "New Width"() -> (w1443:dbl)
            n576 = call "mob_calc_subvi.vi"("Width"=w1443, "Length"=w1442, "Dielectric (d)"=w1441, "Array 2"=w1445, "Array"=w1446) -> ("Vt"=w1439:dbl, "Mobility"=w1444:dbl)  [unwired: 5 in]
            n577 = local write "New Mobility"(w1444) -> ()
            n578 = local write "Array"(w1446) -> ()
            n579 = local write "New Vt"(w1439) -> ()
          }
          event "Slide 2": Value Change {
            n580 = event-data() -> ()  [unwired: 1 in, 5 out]
            n581 = local read "XY Graph 2"() -> (w1465:cluster{dbl[], dbl[]}[])
            n582 = local read "Slide 2"() -> (w1460:dbl)
            n583 = Decimate 1D Array(w1465) -> (w1462:cluster{dbl[], dbl[]}[], w1461:cluster{dbl[], dbl[]}[])
            n584 = local read "NumPts 2"() -> (w1466:dbl)
            n585 = Array To Cluster(array=w1462) -> (cluster=w1470:T4)
            n586 = Unbundle(w1470) -> ("[0]"=w1469:cluster{dbl[], dbl[]})  [unwired: 8 out]
            n587 = Unbundle(w1469) -> (w1468:dbl[], w1467:dbl[])
            n588 = Array Subset(array=w1468, index=w1460, length=w1466) -> (w1458:dbl[])
            n589 = Array Subset(array=w1467, index=w1460, length=w1466) -> (w1457:dbl[])
            n590 = local write "Index 2"(w1460) -> ()
            n591 = Bundle(w1458, w1457) -> (w1464:cluster{dbl[], dbl[]})  [unwired: 1 in]
            n592 = Build Array (concatenate)(w1462, w1461, w1464) -> (w1463:cluster{dbl[], dbl[]}[])
            n593 = local write "XY Graph 2"(w1463) -> ()
            n594 = local write "Array 7"(w1457) -> ()
            n595 = local write "Array 8"(w1458) -> ()
            n596 = call "sts_calc_subvi.vi"("Array 2"=w1458, "Array"=w1457) -> ("STS"=w1459:dbl)  [unwired: 9 in]
            n597 = local write "New S.T.S."(w1459) -> ()
          }
          event "Save Changes?": Mouse Down {
            n598 = event-data() -> ()  [unwired: 1 in, 5 out]
            n599 = flat-sequence {
              tunnel: [w1497] -> w1476
              tunnel: [w1496] -> w1474
              tunnel: [w1496] -> w1473
              tunnel: [w1479] -> w1471
              tunnel: w1476 -> [w1550]
              tunnel: [w1551] -> w1475
              tunnel: w1474 -> [w1551]
              tunnel: w1473 -> [w1549]
              tunnel: [w1547] -> w1472
              tunnel: w1471 -> [w1547]
              tunnel: w1475 -> [w1556]
              tunnel: w1472 -> [w1555]
              frame #0 {
                w1484 = -1
                w1477 = "S.T.S. (V/decade):"
                w1478 = "Threshold V (V):"
                (unwired) 3
                w1482 = 1
                n600 = local read "New Width"() -> (w1510:dbl)
                n601 = local read "New Dielectric"() -> (w1520:dbl)
                n602 = local read "File"() -> (w1497:path)
                n603 = local read "New Length"() -> (w1508:dbl)
                n604 = local read "New Mobility"() -> (w1519:dbl)
                n605 = call-poly <vilib>:"Read From Spreadsheet File.vi"("file path (dialog if empty)"=w1497) -> ("all rows"=w1489:string[][])  [unwired: 6 in, 4 out]
                n606 = Number To Fractional String(number=w1508) -> (F-format string=w1500:string)  [unwired: 3 in]
                n607 = Replace Array Subset(array=w1489, new element=w1500, index (row)=12, index (col)=w1482) -> (w1504:string[][])
                n608 = Number To Fractional String(number=w1510) -> (F-format string=w1511:string)  [unwired: 3 in]
                n609 = Replace Array Subset(array=w1504, new element=w1511, index (row)=13, index (col)=w1482) -> (w1506:string[][])
                n610 = Number To Fractional String(number=w1519) -> (F-format string=w1498:string)  [unwired: 3 in]
                n611 = Number To Fractional String(number=w1520) -> (F-format string=w1499:string)  [unwired: 3 in]
                n612 = Number To Decimal String(number=w1508) -> (decimal integer string=w1507:string)  [unwired: 1 in]
                n613 = Strip Path(path=w1497) -> (stripped path=w1518:path)  [unwired: 1 out]
                n614 = local read "Index"() -> (w1513:string)
                n615 = Replace Array Subset(array=w1506, new element=w1498, index (row)=15, index (col)=w1482) -> (w1505:string[][])
                n616 = Number To Decimal String(number=w1510) -> (decimal integer string=w1509:string)  [unwired: 1 in]
                n617 = Path To String(path=w1518) -> (string=w1516:string)
                n618 = Replace Array Subset(array=w1505, new element=w1499, index (row)=7, index (col)=w1482) -> (w1481:string[][])
                n619 = call "Build Text"("Index"=w1513, "Length"=w1507, "Width"=w1509) -> ("Result"=w1514:string)  [unwired: 11 in, 1 out]
                n620 = Concatenate Strings(w1516, "\\", w1514) -> (w1515:string)
                n621 = String To Path(string=w1515) -> (path=w1496:path)
                n622 = Array Size(array=w1489) -> (size(s)=w1491:i32[])
                n623 = Index Array(array=w1491, index=0) -> (element=w1490:i32)
                n624 = Array Subset(array=w1489, index (row)=0, index (col)=0) -> (w1495:string[][])  [unwired: 2 in]
                n625 = Reshape Array(w1495, w1490) -> (w1483:string[])
                n626 = Search 1D Array(1D array=w1483, element=w1478) -> (index of element=w1487:i32)  [unwired: 1 in]
                n627 = Search 1D Array(1D array=w1483, element=w1477) -> (index of element=w1488:i32)  [unwired: 1 in]
                n628 = Equal?(x=w1487, y=w1484) -> (x = y?=w1485:bool)
                n629 = Equal?(x=w1488, y=w1484) -> (x = y?=w1486:bool)
                n630 = case shown="True" w1485 {
                  tunnel: w1487 -> [_ _]
                  tunnel: w1481 -> [w1537 w1545]
                  tunnel: [w1536 w1544] -> w1480
                  tunnel: w1478 -> [_ w1543]
                  frame False {
                    n631 = local read "New Vt"() -> (w1539:dbl)
                    n632 = Number To Fractional String(number=w1539) -> (F-format string=w1535:string)  [unwired: 3 in]
                    n633 = Replace Array Subset(array=w1537, new element=w1535, index (row)=17, index (col)=1) -> (w1536:string[][])
                  }
                  frame True {
                    n634 = local read "New Vt"() -> (w1546:dbl)
                    n635 = Number To Fractional String(number=w1546) -> (F-format string=w1542:string)  [unwired: 3 in]
                    n636 = Build Array(w1543, w1542) -> (w1541:string[])
                    n637 = Insert Into Array(array=w1545, index (row)=17, new element=w1541) -> (w1544:string[][])  [unwired: 1 in]
                  }
                }
                n638 = case shown="True" w1486 {
                  tunnel: w1488 -> [_ _]
                  tunnel: w1480 -> [w1524 w1532]
                  tunnel: [w1523 w1531] -> w1479
                  tunnel: w1477 -> [_ w1529]
                  frame False {
                    n639 = local read "New S.T.S."() -> (w1526:dbl)
                    n640 = Number To Fractional String(number=w1526) -> (F-format string=w1522:string)  [unwired: 3 in]
                    n641 = Replace Array Subset(array=w1524, new element=w1522, index (row)=18, index (col)=1) -> (w1523:string[][])
                  }
                  frame True {
                    n642 = local read "New S.T.S."() -> (w1533:dbl)
                    n643 = Number To Fractional String(number=w1533) -> (F-format string=w1530:string)  [unwired: 3 in]
                    n644 = Build Array(w1529, w1530) -> (w1528:string[])
                    n645 = Insert Into Array(array=w1532, index (row)=18, new element=w1528) -> (w1531:string[][])  [unwired: 1 in]
                  }
                }
              }
              frame #1 {
                n646 = Equal?(x=w1550, y=w1549) -> (x = y?=w1548:bool)
                n647 = case shown="False" w1548 {
                  tunnel: w1550 -> [w1554 _]
                  tunnel: w1549 -> [w1553 _]
                  frame False {
                    n648 = Move(source path=w1554, 9:TRUE, 10:w1553) -> ()  [unwired: 2 in, 3 out]
                  }
                  frame True {
                  }
                }
              }
              frame #2 {
                n649 = local write "File"(w1556) -> ()
                n650 = call-poly <vilib>:"Write To Spreadsheet File.vi"("2D data"=w1555, "file path (dialog if empty)"=w1556) -> ()  [unwired: 6 in, 1 out]
              }
            }
          }
          event "Save Changes? 2": Mouse Down {
            n651 = event-data() -> ()  [unwired: 1 in, 5 out]
            n652 = stacked-sequence {
              seq-local: [w1577 _ _ _ _] -> [_ w1630 _ _ _]
              seq-local: [w1576 _ _ _ _] -> [_ w1631 _ _ _]
              seq-local: [w1576 _ _ _ _] -> [_ w1629 _ _ _]
              seq-local: [w1559 _ _ _ _] -> [_ w1627 _ _ _]
              seq-local: [_ w1631 _ _ _] -> [_ _ w1636 _ _]
              seq-local: [_ w1627 _ _ _] -> [_ _ w1635 _ _]
              frame #0 {
                w1564 = -1
                w1557 = "S.T.S. (V/decade):"
                w1558 = "Threshold V (V):"
                (unwired) 3
                w1562 = 1
                n653 = local read "New Width"() -> (w1590:dbl)
                n654 = local read "New Dielectric"() -> (w1600:dbl)
                n655 = local read "File"() -> (w1577:path)
                n656 = local read "New Length"() -> (w1588:dbl)
                n657 = local read "New Mobility"() -> (w1599:dbl)
                n658 = call-poly <vilib>:"Read From Spreadsheet File.vi"("file path (dialog if empty)"=w1577) -> ("all rows"=w1569:string[][])  [unwired: 6 in, 4 out]
                n659 = Number To Fractional String(number=w1588) -> (F-format string=w1580:string)  [unwired: 3 in]
                n660 = Replace Array Subset(array=w1569, new element=w1580, index (row)=12, index (col)=w1562) -> (w1584:string[][])
                n661 = Number To Fractional String(number=w1590) -> (F-format string=w1591:string)  [unwired: 3 in]
                n662 = Replace Array Subset(array=w1584, new element=w1591, index (row)=13, index (col)=w1562) -> (w1586:string[][])
                n663 = Number To Fractional String(number=w1599) -> (F-format string=w1578:string)  [unwired: 3 in]
                n664 = Number To Fractional String(number=w1600) -> (F-format string=w1579:string)  [unwired: 3 in]
                n665 = Number To Decimal String(number=w1588) -> (decimal integer string=w1587:string)  [unwired: 1 in]
                n666 = Strip Path(path=w1577) -> (stripped path=w1598:path)  [unwired: 1 out]
                n667 = local read "Index"() -> (w1593:string)
                n668 = Replace Array Subset(array=w1586, new element=w1578, index (row)=15, index (col)=w1562) -> (w1585:string[][])
                n669 = Number To Decimal String(number=w1590) -> (decimal integer string=w1589:string)  [unwired: 1 in]
                n670 = Path To String(path=w1598) -> (string=w1596:string)
                n671 = Replace Array Subset(array=w1585, new element=w1579, index (row)=7, index (col)=w1562) -> (w1561:string[][])
                n672 = call "Build Text2"("Index"=w1593, "Length"=w1587, "Width"=w1589) -> ("Result"=w1594:string)  [unwired: 11 in, 1 out]
                n673 = Concatenate Strings(w1596, "\\", w1594) -> (w1595:string)
                n674 = String To Path(string=w1595) -> (path=w1576:path)
                n675 = Array Size(array=w1569) -> (size(s)=w1571:i32[])
                n676 = Index Array(array=w1571, index=0) -> (element=w1570:i32)
                n677 = Array Subset(array=w1569, index (row)=0, index (col)=0) -> (w1575:string[][])  [unwired: 2 in]
                n678 = Reshape Array(w1575, w1570) -> (w1563:string[])
                n679 = Search 1D Array(1D array=w1563, element=w1558) -> (index of element=w1567:i32)  [unwired: 1 in]
                n680 = Search 1D Array(1D array=w1563, element=w1557) -> (index of element=w1568:i32)  [unwired: 1 in]
                n681 = Equal?(x=w1567, y=w1564) -> (x = y?=w1565:bool)
                n682 = Equal?(x=w1568, y=w1564) -> (x = y?=w1566:bool)
                n683 = case shown="True" w1565 {
                  tunnel: w1567 -> [_ _]
                  tunnel: w1561 -> [w1617 w1625]
                  tunnel: [w1616 w1624] -> w1560
                  tunnel: w1558 -> [_ w1623]
                  frame False {
                    n684 = local read "New Vt"() -> (w1619:dbl)
                    n685 = Number To Fractional String(number=w1619) -> (F-format string=w1615:string)  [unwired: 3 in]
                    n686 = Replace Array Subset(array=w1617, new element=w1615, index (row)=17, index (col)=1) -> (w1616:string[][])
                  }
                  frame True {
                    n687 = local read "New Vt"() -> (w1626:dbl)
                    n688 = Number To Fractional String(number=w1626) -> (F-format string=w1622:string)  [unwired: 3 in]
                    n689 = Build Array(w1623, w1622) -> (w1621:string[])
                    n690 = Insert Into Array(array=w1625, index (row)=17, new element=w1621) -> (w1624:string[][])  [unwired: 1 in]
                  }
                }
                n691 = case shown="True" w1566 {
                  tunnel: w1568 -> [_ _]
                  tunnel: w1560 -> [w1604 w1612]
                  tunnel: [w1603 w1611] -> w1559
                  tunnel: w1557 -> [_ w1609]
                  frame False {
                    n692 = local read "New S.T.S."() -> (w1606:dbl)
                    n693 = Number To Fractional String(number=w1606) -> (F-format string=w1602:string)  [unwired: 3 in]
                    n694 = Replace Array Subset(array=w1604, new element=w1602, index (row)=18, index (col)=1) -> (w1603:string[][])
                  }
                  frame True {
                    n695 = local read "New S.T.S."() -> (w1613:dbl)
                    n696 = Number To Fractional String(number=w1613) -> (F-format string=w1610:string)  [unwired: 3 in]
                    n697 = Build Array(w1609, w1610) -> (w1608:string[])
                    n698 = Insert Into Array(array=w1612, index (row)=18, new element=w1608) -> (w1611:string[][])  [unwired: 1 in]
                  }
                }
              }
              frame #1 {
                n699 = Equal?(x=w1630, y=w1629) -> (x = y?=w1628:bool)
                n700 = case shown="False" w1628 {
                  tunnel: w1630 -> [w1634 _]
                  tunnel: w1629 -> [w1633 _]
                  frame False {
                    n701 = Move(source path=w1634, 9:TRUE, 10:w1633) -> ()  [unwired: 2 in, 3 out]
                  }
                  frame True {
                  }
                }
              }
              frame #2 {
                n702 = local write "File"(w1636) -> ()
                n703 = call-poly <vilib>:"Write To Spreadsheet File.vi"("2D data"=w1635, "file path (dialog if empty)"=w1636) -> ()  [unwired: 6 in, 1 out]
              }
              frame #3 {
                w1700 = 0
                n704 = local read "NumPts 2"() -> (w1659:dbl)
                n705 = local read "NumPts"() -> (w1666:dbl)
                n706 = local read "Row Start"() -> (w1665:dbl)
                n707 = local read "File"() -> (w1705:path)
                n708 = property on="Image Out" class="ImageControl"() -> (error out=w1640:errorcluster, "Image Center Position"=w1644:cluster{"X":u32, "Y":u32})  [unwired: 2 in, 1 out]
                n709 = Strip Path(path=w1705) -> (stripped path=w1696:path, name=w1718:string)
                n710 = local write "Folder"(w1696) -> ()
                n711 = List Folder(path=w1696) -> (filenames=w1711:string[])  [unwired: 3 in, 3 out]
                n712 = Unbundle(w1644) -> ("X"=w1642:u32)  [unwired: 1 out]
                n713 = Array Size(array=w1711) -> (size(s)=w1706:i32)
                n714 = Path To String(path=w1696) -> (string=w1719:string)
                n715 = Search 1D Array(1D array=w1711, element=w1718) -> (index of element=w1708:i32)  [unwired: 1 in]
                n716 = Bundle("X"=w1642, 0) -> (w1643:cluster{"X":u32, i32})  [unwired: 1 in]
                n717 = Decrement(x=w1706) -> (x-1=w1709:i32)
                n718 = Equal?(x=w1708, y=w1709) -> (x = y?=w1710:bool)
                n719 = case shown="False" w1710 {
                  tunnel: w1708 -> [w1841 _]
                  tunnel: [w1840 0] -> w1707
                  frame False {
                    n720 = Increment(x=w1841) -> (x+1=w1840:i32)
                  }
                  frame True {
                  }
                }
                n721 = Index Array(array=w1711, index=w1707) -> (element=w1712:string)
                n722 = local write "Data Name"(w1712) -> ()
                n723 = Concatenate Strings(w1719, "\\", w1712) -> (w1717:string)
                n724 = property on="Image Out" class="ImageControl"(error in=w1640, "Image Center Position"=w1643) -> ()  [unwired: 1 in, 2 out]
                n725 = String To Path(string=w1717) -> (path=w1667:path)
                n726 = call "sub_thresh_swing_subvi.vi"("Path"=w1667, "NumPts"=w1659, "Row Start"=w1665) -> ("Index"=w1660:dbl, "XY Graph"=w1655:cluster{dbl[], dbl[]}[], "Sub Threshold Swing"=w1668:dbl)  [unwired: 8 in, 2 out]
                n727 = Decimate 1D Array(w1655) -> (w1658:cluster{dbl[], dbl[]}[])  [unwired: 1 out]
                n728 = Array To Cluster(array=w1658) -> (cluster=w1656:T4)
                n729 = Unbundle(w1656) -> ("[0]"=w1657:cluster{dbl[], dbl[]})  [unwired: 8 out]
                n730 = Unbundle(w1657) -> (w1654:dbl[], w1653:dbl[])
                n731 = local write "S.T.S."(w1668) -> ()
                n732 = local write "XY Graph 2"(w1655) -> ()
                n733 = local write "Index 2"(w1660) -> ()
                n734 = call "mobility_subvi.vi"("Path"=w1667, "NumPts"=w1666, "Row Start"=w1665) -> ("Dielectric (d)"=w1671:dbl, "Index"=w1676:dbl, "XY Graph"=w1679:cluster{dbl[], dbl[]}[], "Length"=w1669:dbl, "Vt"=w1672:dbl, "Width"=w1670:dbl, "Table Control"=w1715:string[][], "Table Control 2"=w1714:string[][], "Recorded"=w1652:cluster{"Vt":dbl, "STS":dbl, "On/Off":dbl}, "Mobility"=w1713:dbl)  [unwired: 3 in]
                n735 = local write "Dielectric (d)"(w1671) -> ()
                n736 = local write "Threshold V"(w1672) -> ()
                n737 = local write "New Dielectric"(w1671) -> ()
                n738 = Decimate 1D Array(w1679) -> (w1680:cluster{dbl[], dbl[]}[])  [unwired: 1 out]
                n739 = Array To Cluster(array=w1680) -> (cluster=w1682:T4)
                n740 = local write "Table Control"(w1715) -> ()
                n741 = Unbundle(w1682) -> ("[0]"=w1681:cluster{dbl[], dbl[]})  [unwired: 8 out]
                n742 = Unbundle(w1681) -> (w1662:dbl[], w1661:dbl[])
                n743 = local write "XY Graph"(w1679) -> ()
                n744 = local write "Table Control 2"(w1714) -> ()
                n745 = local write "Mobility"(w1713) -> ()
                n746 = Array Subset(array=w1662, index=w1676, length=w1666) -> (w1678:dbl[])
                n747 = Array Subset(array=w1661, index=w1676, length=w1666) -> (w1677:dbl[])
                n748 = local write "Width"(w1670) -> ()
                n749 = local write "Length"(w1669) -> ()
                n750 = local write "Array 2"(w1677) -> ()
                n751 = Unbundle(w1652) -> ("Vt"=w1651:dbl, "STS"=w1650:dbl, "On/Off"=w1649:dbl)
                n752 = local write "On/Off"(w1649) -> ()
                n753 = local write "Array"(w1678) -> ()
                n754 = local write "Slide"(w1676) -> ()
                n755 = local write "Index"(w1676) -> ()
                n756 = local write "STS recorded"(w1650) -> ()
                n757 = local write "Vt recorded"(w1651) -> ()
                n758 = Array Subset(array=w1654, index=w1660, length=w1659) -> (w1664:dbl[])
                n759 = Array Subset(array=w1653, index=w1660, length=w1659) -> (w1663:dbl[])
                n760 = local write "New Width"(w1670) -> ()
                n761 = local write "New Length"(w1669) -> ()
                n762 = local write "File"(w1667) -> ()
                n763 = local write "Array 8"(w1664) -> ()
                n764 = local write "Array 7"(w1663) -> ()
                n765 = call-poly <vilib>:"Read From Spreadsheet File.vi"("file path (dialog if empty)"=w1667) -> ("all rows"=w1702:string[][])  [unwired: 6 in, 4 out]
                n766 = Array Size(array=w1702) -> (size(s)=w1701:i32[])
                n767 = local read "Folder"() -> (w1690:path)
                n768 = List Folder(path=w1690) -> (filenames=w1695:string[])  [unwired: 3 in, 3 out]
                n769 = Index Array(array=w1701, index=w1700) -> (element=w1674:i32)
                n770 = Subtract(x=w1674, y=20) -> (x-y=w1673:i32)
                n771 = property on="Slide" class="Slide (strict)"("Scale.Maximum"=w1673) -> ()  [unwired: 2 in, 2 out]
                n772 = Array Subset(array=w1702, index (row)=w1700, index (col)=w1700, length (col)=3) -> (w1703:string[][])  [unwired: 1 in]
                n773 = Reshape Array(w1703, w1674) -> (w1683:string[])
                n774 = Search 1D Array(1D array=w1683, element="Mobility (cm^2/Vs):") -> (index of element=w1688:i32)  [unwired: 1 in]
                n775 = Search 1D Array(1D array=w1683, element="Index:") -> (index of element=w1697:i32)  [unwired: 1 in]
                n776 = Increment(x=w1697) -> (x+1=w1698:i32)
                n777 = Index Array(array=w1683, index=w1698) -> (element=w1693:string)
                n778 = while {
                  tunnel: w1695 -> [w1727]
                  tunnel: w1693 -> [w1725]
                  tunnel: [w1724] -> _
                  tunnel: [w1724] -> w1694
                  tunnel: w1674 -> [w1723]
                  i -> [w1724]
                  stop <- w1720 stop-if-true
                  n779 = Index Array(array=w1727, index=w1724) -> (element=w1728:string)
                  n780 = xnode "Match Regular Expression"("input string"=w1728, "regular expression"=w1725) -> ("whole match"=w1726:string)  [unwired: 4 in, 4 out]
                  n781 = Equal?(x=w1726, y=w1725) -> (x = y?=w1722:bool)
                  n782 = Equal?(x=w1723, y=w1724) -> (x = y?=w1721:bool)
                  n783 = Or(x=w1722, y=w1721) -> (x .or. y?=w1720:bool)
                }
                n784 = local write "Index"(w1693) -> ()
                n785 = Increment(x=w1688) -> (x+1=w1687:i32)
                n786 = local read "No Image"() -> (w1645:path)
                n787 = Index Array(array=w1683, index=w1687) -> (element=w1685:string)
                n788 = Fract/Exp String To Number(string=w1685) -> (number=w1684:dbl)  [unwired: 3 in, 1 out]
                n789 = local write "Recorded Mobility"(w1684) -> ()
                n790 = Path To String(path=w1690) -> (string=w1692:string)
                n791 = local read "Image Out"() -> (w1637:T1)
                n792 = Index Array(array=w1695, index=w1694) -> (element=w1647:string)
                n793 = Empty String/Path?(string/path=w1647) -> (empty?=w1648:bool)
                n794 = Concatenate Strings(w1692, "\\", w1647) -> (w1691:string)
                n795 = local write "Image Name"(w1647) -> ()
                n796 = String To Path(string=w1691) -> (path=w1646:path)
                n797 = Select(t=w1645, s=w1648, f=w1646) -> (s? t:f=w1639:path)
                n798 = local write "File"(w1639) -> ()
                n799 = call "IMAQ ReadFile"("File Path"=w1639, "Image"=w1637) -> ("Image Out"=w1638:T1)  [unwired: 5 in, 4 out]
                n800 = local write "Image Out 2"(w1638) -> ()
                n801 = local write "Image Out"(w1638) -> ()
                n802 = invoke on="Image Out" class="ImageControl" method="Clear ROI"() -> ()  [unwired: 3 in, 3 out]
              }
              frame #4 {
                n803 = local read "Folder"() -> (w1843:path)
                n804 = Build Path(base path=w1843, name or relative path="ROI") -> (appended path=w1845:path)
                n805 = local read "Index"() -> (w1844:string)
                n806 = Build Path(base path=w1845, name or relative path=w1844) -> (appended path=w1850:path)
                n807 = invoke on="Image Out" class="ImageControl" method="Clear ROI"() -> (error out=w1849:errorcluster)  [unwired: 3 in, 2 out]
                n808 = call <vilib>:"Check if File or Folder Exists.vi"("error in (no error)"=w1849, "path"=w1850) -> ("file or folder exists?"=w1847:bool, "dup path"=w1848:path)  [unwired: 7 in, 1 out]
                n809 = case shown="True" w1847 {
                  tunnel: w1848 -> [_ w1851]
                  frame False {
                  }
                  frame True {
                    n810 = Read from Text File(file (use dialog)=w1851) -> (text=w1855:string)  [unwired: 3 in, 3 out]
                    n811 = property on="Image Out" class="ImageControl"() -> ("ROI"=w1852:T5)  [unwired: 2 in, 2 out]
                    n812 = Unflatten From String(type=w1852, binary string=w1855) -> (value=w1853:T5, error out=w1854:errorcluster)  [unwired: 3 in, 1 out]
                    n813 = property on="Image Out" class="ImageControl"(error in=w1854, "ROI"=w1853) -> ()  [unwired: 1 in, 2 out]
                  }
                }
              }
            }
          }
          event "Export": Mouse Down {
            n814 = event-data() -> ()  [unwired: 1 in, 7 out]
            n815 = call "OA_ConnectToOrigin.vi"() -> ("error out"=w1877:errorcluster, "Origin.IOApplication"=w1878:refnum<k7>)  [unwired: 8 in]
            n816 = local read "Folder"() -> (w1874:path)
            n817 = local read "Project"() -> (w1876:path)
            n818 = call "OA_Load.vi"("error in (no error)"=w1877, "Path"=w1876, "Origin.IOApplication"=w1878) -> ("error out"=w1868:errorcluster, "Origin.IOApplication"=w1869:refnum<k7>)  [unwired: 1 out]
            n819 = call "OAExecute.vi"("script"="document -m 3;", "Error IO"=w1868, "Origin.IOApplication"=w1869) -> ("Error IO Out"=w1866:errorcluster, "Origin.IOApplication"=w1867:refnum<k7>)  [unwired: 1 in, 1 out]
            n820 = flat-sequence {
              tunnel: w1874 -> [w1898]
              tunnel: w1875 -> [w1897]
              tunnel: [w1887] -> w1880
              tunnel: [w1888] -> w1879
              tunnel: w1867 -> [w1892]
              tunnel: w1866 -> [w1891]
              tunnel: w1874 -> [w1914]
              tunnel: w1875 -> [w1913]
              tunnel: w1880 -> [w1909]
              tunnel: w1879 -> [w1910]
              tunnel: [w1904] -> w1873
              tunnel: [w1903] -> w1872
              tunnel: w1874 -> [w1925]
              tunnel: w1875 -> [w1924]
              tunnel: w1873 -> [w1920]
              tunnel: w1872 -> [w1919]
              tunnel: [w1918] -> w1871
              tunnel: [w1917] -> w1870
              tunnel: w1874 -> [w1940]
              tunnel: w1875 -> [w1939]
              tunnel: w1871 -> [w1934]
              tunnel: w1870 -> [w1933]
              tunnel: [w1931] -> w1864
              tunnel: [w1930] -> w1863
              frame #0 {
                n821 = call "Param_Analysis.vi"("error in (no error)"=w1891, "Folder 2"=w1898, "Parameter String"="Mobility (cm^2/Vs):", "Parameter Name"="Mobility", "Folder"=w1897) -> ("error out"=w1894:errorcluster, "Array 4"=w1884:string[], "Array 3"=w1893:string[][])  [unwired: 3 in, 1 out]
                n822 = call "Origin_Export.vi"("String 3"="[MobHistTab]Sheet1", "error in (no error)"=w1894, "Array"=w1893, "String 2"="[MOBvsLTable]Mobilities", "String"="pe_cd \"Mobility Chart\";", "Origin.IOApplication"=w1892, "Array 2"=w1884) -> ("reference out"=w1890:refnum<k7>, "error out"=w1889:errorcluster)  [unwired: 2 in, 1 out]
                n823 = call "OAExecute.vi"("script"="window -a MOBvsLTable;\nwindow -s TV;", "Error IO"=w1889, "Origin.IOApplication"=w1890) -> ("Error IO Out"=w1887:errorcluster, "Origin.IOApplication"=w1888:refnum<k7>)  [unwired: 1 in, 1 out]
              }
              frame #1 {
                n824 = call "Param_Analysis.vi"("error in (no error)"=w1909, "Folder 2"=w1914, "Parameter String"="On/Off Current:", "Parameter Name"="On_Off_Current", "Folder"=w1913) -> ("error out"=w1908:errorcluster, "Array 4"=w1902:string[], "Array 3"=w1905:string[][])  [unwired: 3 in, 1 out]
                n825 = call "Origin_Export.vi"("String 3"="[OnOffHistTab]Sheet1", "error in (no error)"=w1908, "Array"=w1905, "String 2"="[OnOffTable]On/Off Ratios", "String"="pe_cd \"OnOff vs L\";", "Origin.IOApplication"=w1910, "Array 2"=w1902) -> ("reference out"=w1904:refnum<k7>, "error out"=w1903:errorcluster)  [unwired: 2 in, 1 out]
              }
              frame #2 {
                n826 = call "Param_Analysis.vi"("Folder 2"=w1925, "Parameter String"="S.T.S. (V/decade):", "Parameter Name"="STS", "Folder"=w1924) -> ("Array 4"=w1916:string[], "Array 3"=w1921:string[][])  [unwired: 4 in, 2 out]
                n827 = call "Origin_Export.vi"("String 3"="[SHistTab]Sheet1", "error in (no error)"=w1919, "Array"=w1921, "String 2"="[STable]Threshold Swing", "String"="pe_cd \"Threshold Swing vs L\";", "Origin.IOApplication"=w1920, "Array 2"=w1916) -> ("reference out"=w1917:refnum<k7>, "error out"=w1918:errorcluster)  [unwired: 2 in, 1 out]
              }
              frame #3 {
                n828 = call "Param_Analysis.vi"("Folder 2"=w1940, "Parameter String"="Threshold V (V):", "Parameter Name"="Threshold_V", "Folder"=w1939) -> ("Array 4"=w1929:string[], "Array 3"=w1932:string[][])  [unwired: 4 in, 2 out]
                n829 = call "Origin_Export.vi"("String 3"="[VtHistTab]Sheet1", "error in (no error)"=w1934, "Array"=w1932, "String 2"="[VtTable]Threshold Voltages", "String"="pe_cd \"Threshold Voltage vs L\";", "Origin.IOApplication"=w1933, "Array 2"=w1929) -> ("reference out"=w1931:refnum<k7>, "error out"=w1930:errorcluster)  [unwired: 2 in, 1 out]
              }
            }
            n830 = Build Path(base path=w1874, name or relative path="Stats") -> (appended path=w1859:path)
            n831 = call <vilib>:"Check if File or Folder Exists.vi"("path"=w1859) -> ("file or folder exists?"=w1882:bool, "dup path"=w1881:path)  [unwired: 8 in, 1 out]
            n832 = case shown="False" w1882 {
              tunnel: w1881 -> [w1942 w1943]
              tunnel: [w1941 w1943] -> w1875
              frame False {
                n833 = Create Folder(path (use dialog)=w1942) -> (created path=w1941:path)  [unwired: 2 in, 2 out]
              }
              frame True {
              }
            }
            n834 = call "File Dialog"("start path"=w1859) -> ("selected path"=w1858:path)  [unwired: 11 in, 3 out]
            n835 = Path To String(path=w1858) -> (string=w1857:string)
            n836 = call "OAExecute.vi"("script"="pe_cd /;\npe_cd \"Mobility Chart\"; ", "Error IO"=w1863, "Origin.IOApplication"=w1864) -> ("Error IO Out"=w1860:errorcluster, "Origin.IOApplication"=w1861:refnum<k7>)  [unwired: 1 in, 1 out]
            n837 = call "OASaveProject.vi"("path"=w1857, "Error IO"=w1860, "Origin.IOApplication"=w1861) -> ()  [unwired: 3 out]
          }
          event "Blank Button": Mouse Down {
            n838 = event-data() -> ()  [unwired: 1 in, 7 out]
            n839 = local read "File"() -> (w1951:path)
            n840 = Strip Path(path=w1951) -> (stripped path=w1947:path, name=w1949:string)
            n841 = Path To String(path=w1947) -> (string=w1946:string)
            n842 = Concatenate Strings(w1946, "\\", "X_", w1949) -> (w1945:string)
            n843 = String To Path(string=w1945) -> (path=w1944:path)
            n844 = Move(source path=w1951, 10:w1944) -> ()  [unwired: 3 in, 3 out]
            n845 = local write "File"(w1944) -> ()
          }
          event "Cancel Button": Mouse Down {
            (unwired) 6
            n846 = event-data() -> ()  [unwired: 1 in, 7 out]
            n847 = call "Simulate_Keyboard.vi"("Action"=2, "Virtual Key"=162) -> ()  [unwired: 7 in, 1 out]
          }
        }
        n848 = property on="Image Out" class="ImageControl"() -> ("ROI"=w363:T5)  [unwired: 2 in, 2 out]
        n849 = local read "Image Out"() -> (w392:T1)
        n850 = property on="Image Out" class="ImageControl"() -> ("ZoomSingle"=w406:cluster{"X":sgl, "Y":sgl})  [unwired: 2 in, 2 out]
        n851 = property on="Image Out" class="ImageControl"() -> ("Bounds"=w407:T6)  [unwired: 2 in, 2 out]
        n852 = Unbundle By Name(w363) -> ("Contours"=w437:T7)
        n853 = call <vilib>:"Intialize Keyboard.vi"() -> ("device ID"=w418:refnum<k1>)  [unwired: 10 in, 1 out]
        n854 = property on="Image Out" class="ImageControl"() -> ("Image Center Position"=w413:cluster{"X":u32, "Y":u32})  [unwired: 2 in, 2 out]
        n855 = call "IMAQ Clear Overlay"("Image"=w392) -> ("Image Out"=w391:T1)  [unwired: 9 in, 1 out]
        n856 = call-poly <vilib>:"Acquire Input Data.vi"("device ID"=w418) -> ("keys pressed"=w417:T8)  [unwired: 16 in, 2 out]
        n857 = Initialize Array(0) -> (w435:i32[])  [unwired: 1 in]
        n858 = local read "Magnification"() -> (w426:u16)
        n859 = Unbundle(w407) -> ("Width"=w404:u32, "Height"=w403:u32)
        n860 = Array Size(array=w437) -> (size(s)=w436:i32)
        n861 = Unbundle(w406) -> ("X"=w381:sgl, "Y"=w405:sgl)
        n862 = event shown="[2] \" Folder\": Value Change" {
          selector: _ -> [_ _ _ _ _ _ _]
          dyn-events: _ -> [_ _ _ _ _ _ _]
          timeout: 10 -> [_ _ _ _ _ _ _]
          event "Remove Button": Mouse Down {
            w443 = 0
            n863 = property on="Image Out" class="ImageControl"() -> ("ROI"=w441:T5)  [unwired: 2 in, 2 out]
            n864 = event-data() -> ()  [unwired: 1 in, 7 out]
            n865 = Unbundle(w441) -> ("Global Rectangle"=w444:i32[], "Contours"=w446:T7)
            n866 = Reverse 1D Array(array=w444) -> (reversed array=w445:i32[])
            n867 = Reverse 1D Array(array=w446) -> (reversed array=w447:T7)
            n868 = Delete From Array(array=w445, index=w443) -> (array with subset deleted=w448:i32[])  [unwired: 1 in, 1 out]
            n869 = Delete From Array(array=w447, index=w443) -> (array with subset deleted=w449:T7)  [unwired: 1 in, 1 out]
            n870 = Reverse 1D Array(array=w448) -> (reversed array=w450:i32[])
            n871 = Reverse 1D Array(array=w449) -> (reversed array=w451:T7)
            n872 = Bundle(w450, w451) -> (w442:T9)  [unwired: 1 in]
            n873 = local write "ROI Descriptor out"(w441) -> ()
            n874 = local write "ROI Descriptor"(w442) -> ()
            n875 = property on="Image Out" class="ImageControl"("ROI"=w442) -> ()  [unwired: 2 in, 2 out]
          }
          event "Undo Button": Mouse Down {
            n876 = event-data() -> ()  [unwired: 1 in, 7 out]
            n877 = invoke on="Image Out" class="ImageControl" method="Clear ROI"() -> ()  [unwired: 3 in, 3 out]
          }
          event "Folder": Value Change {
            n878 = event-data() -> ()  [unwired: 1 in, 5 out]
            n879 = local read "File"() -> (w453:path)
            n880 = call "Vision Acquisition"("Image Path"=w453) -> ("Image Out"=w452:T1)  [unwired: 25 in, 1 out]
            n881 = local write "Image Out 2"(w452) -> ()
            n882 = local write "Image Out"(w452) -> ()
            n883 = invoke on="Image Out" class="ImageControl" method="Clear ROI"() -> ()  [unwired: 3 in, 3 out]
          }
          event "Zoom": Value Change {
            n884 = event-data() -> ()  [unwired: 1 in, 5 out]
            n885 = local read "Zoom"() -> (w454:i16)
            n886 = Bundle("Zoom"=w454, "Zoom"=w454) -> (w455:cluster{"Zoom":i16, "Zoom":i16})  [unwired: 1 in]
            n887 = property on="Image Out" class="ImageControl"("ZoomInteger"=w455) -> ()  [unwired: 2 in, 2 out]
          }
          event Timeout {
            n888 = event-data() -> ()  [unwired: 1 in, 2 out]
          }
          event "Image Out": Mouse Enter {
            (unwired) 6
            n889 = event-data() -> ()  [unwired: 1 in, 3 out]
            n890 = call "Simulate_Keyboard.vi"("Action"=0, "Virtual Key"=162) -> ()  [unwired: 7 in, 1 out]
          }
          event "Image Out": Mouse Leave {
            n891 = event-data() -> ()  [unwired: 1 in, 3 out]
            n892 = flat-sequence {
              frame #0 {
                n893 = Wait (ms)(milliseconds to wait=10) -> ()  [unwired: 1 out]
              }
              frame #1 {
                (unwired) 6
                n894 = call "Simulate_Keyboard.vi"("Action"=2, "Virtual Key"=162) -> ()  [unwired: 7 in, 1 out]
              }
            }
          }
        }
        n895 = Build Array(0.505025, 0.252522, 0.127742, 0.050345, 0.031129) -> (w427:dbl[])
        n896 = Index Array(array=w417) -> (element=w421:T10)  [unwired: 1 in]
        n897 = Divide(x=w404, y=w381) -> (x/y=w394:sgl)
        n898 = Multiply(x=w394, y=0.5) -> (x*y=w400:dbl)
        n899 = Divide(x=w403, y=w405) -> (x/y=w393:sgl)
        n900 = Multiply(x=w393, y=0.5) -> (x*y=w399:dbl)
        n901 = Array Subset(array=w427, index=w426, length=1) -> (w424:dbl[])
        n902 = property on="Image Out" class="ImageControl"() -> ("ZoomInteger"=w416:cluster{"X":i32, "Y":i32})  [unwired: 2 in, 2 out]
        n903 = Unbundle(w413) -> ("X"=w395:u32, "Y"=w396:u32)
        n904 = Subtract(x=w396, y=w399) -> (x-y=w397:dbl)
        n905 = Subtract(x=w395, y=w400) -> (x-y=w398:dbl)
        n906 = Add(x=w398, y=w394) -> (x+y=w412:dbl)
        n907 = Add(x=w397, y=w393) -> (x+y=w411:dbl)
        n908 = To Double Precision Float(number=w424) -> (double precision float=w423:dbl[])
        n909 = local write "ROI Descriptor"(w363) -> ()
        n910 = Reciprocal(x=w381) -> (1/x=w380:sgl)
        n911 = Unbundle(w416) -> ("X"=w415:i32)  [unwired: 1 out]
        n912 = Multiply(x=w380, y=10) -> (x*y=w382:sgl)
        n913 = case shown="\"EQUALS\"" w421 {
          tunnel: w395 -> [w462 w468 w472 w474 w478 w480 w482 w484 w486 w488 w490 w492 w494 w496 w498 w500 w502 w504 w506 w508 w510 w512 w514 w516 w518 w520 w522 w524 w526 w528 w530 w532 w534 w536 w538 w540 w542 w544 w546 w548 w550 w552 w554 w556 w558 w560 w562 w564 w566 w568 w570 w572 w574 w576 w578 w580 w582 w584 w586 w588 w590 w592 w594 w596 w598 w600 w602 w604 w606 w608 w610 w612 w614 w616 w618 w620 w622 w624 w626 w628 w630 w632 w634 w636 w638 w640 w642 w644 w646 w648 w650 w652 w654 w656 w658 w660 w662 w664 w666 w668 w670 w672 w674 w676 w678]
          tunnel: [w462 w467 w471 w474 w478 w480 w482 w484 w486 w488 w490 w492 w494 w496 w498 w500 w502 w504 w506 w508 w510 w512 w514 w516 w518 w520 w522 w524 w526 w528 w530 w532 w534 w536 w538 w540 w542 w544 w546 w548 w550 w552 w554 w556 w558 w560 w562 w564 w566 w568 w570 w572 w574 w576 w578 w580 w582 w584 w586 w588 w590 w592 w594 w596 w598 w600 w602 w604 w606 w608 w610 w612 w614 w616 w618 w620 w622 w624 w626 w628 w630 w632 w634 w636 w638 w640 w642 w644 w646 w648 w650 w652 w654 w656 w658 w660 w662 w664 w666 w668 w670 w672 w674 w676 w678] -> w420
          tunnel: w396 -> [w464 w466 w470 w476 w477 w479 w481 w483 w485 w487 w489 w491 w493 w495 w497 w499 w501 w503 w505 w507 w509 w511 w513 w515 w517 w519 w521 w523 w525 w527 w529 w531 w533 w535 w537 w539 w541 w543 w545 w547 w549 w551 w553 w555 w557 w559 w561 w563 w565 w567 w569 w571 w573 w575 w577 w579 w581 w583 w585 w587 w589 w591 w593 w595 w597 w599 w601 w603 w605 w607 w609 w611 w613 w615 w617 w619 w621 w623 w625 w627 w629 w631 w633 w635 w637 w639 w641 w643 w645 w647 w649 w651 w653 w655 w657 w659 w661 w663 w665 w667 w669 w671 w673 w675 w677]
          tunnel: [w463 w466 w470 w475 w477 w479 w481 w483 w485 w487 w489 w491 w493 w495 w497 w499 w501 w503 w505 w507 w509 w511 w513 w515 w517 w519 w521 w523 w525 w527 w529 w531 w533 w535 w537 w539 w541 w543 w545 w547 w549 w551 w553 w555 w557 w559 w561 w563 w565 w567 w569 w571 w573 w575 w577 w579 w581 w583 w585 w587 w589 w591 w593 w595 w597 w599 w601 w603 w605 w607 w609 w611 w613 w615 w617 w619 w621 w623 w625 w627 w629 w631 w633 w635 w637 w639 w641 w643 w645 w647 w649 w651 w653 w655 w657 w659 w661 w663 w665 w667 w669 w671 w673 w675 w677] -> w419
          tunnel: w382 -> [w461 w465 w469 w473 _ _ _ _ _ _ _ _ _ _ _ _ _ _ _ _ _ _ _ _ _ _ _ _ _ _ _ _ _ _ _ _ _ _ _ _ _ _ _ _ _ _ _ _ _ _ _ _ _ _ _ _ _ _ _ _ _ _ _ _ _ _ _ _ _ _ _ _ _ _ _ _ _ _ _ _ _ _ _ _ _ _ _ _ _ _ _ _ _ _ _ _ _ _ _ _ _ _ _ _ _]
          frame "DOWN" {
            n914 = Add(x=w464, y=w461) -> (x+y=w463:sgl)
          }
          frame "LEFT" {
            n915 = Subtract(x=w468, y=w465) -> (x-y=w467:sgl)
          }
          frame "RIGHT" {
            n916 = Add(x=w472, y=w469) -> (x+y=w471:sgl)
          }
          frame "UP" {
            n917 = Subtract(x=w476, y=w473) -> (x-y=w475:sgl)
          }
          frame "ENTER (num pad)" {
          }
          frame "' (quote)" {
          }
          frame "END" {
          }
          frame "EQUALS" {
          }
          frame "ESCAPE" {
          }
          frame "GRAVE (`)" {
          }
          frame "HOME" {
          }
          frame "INSERT" {
          }
          frame "LBRACKET" {
          }
          frame "LCONTROL" {
          }
          frame "L ALT" {
          }
          frame "LSHIFT" {
          }
          frame "LWIN" {
          }
          frame "MINUS" {
          }
          frame "MULTIPLY" {
          }
          frame "NEXT" {
          }
          frame "NUMLOCK" {
          }
          frame "NUMPAD_0" {
          }
          frame "NUMPAD_1" {
          }
          frame "NUMPAD_2" {
          }
          frame "NUMPAD_3" {
          }
          frame "NUMPAD_4" {
          }
          frame "NUMPAD_5" {
          }
          frame "NUMPAD_6" {
          }
          frame "NUMPAD_7" {
          }
          frame "NUMPAD_8" {
          }
          frame "NUMPAD_9" {
          }
          frame "PAUSE" {
          }
          frame "PERIOD" {
          }
          frame "PRIOR (PG UP)" {
          }
          frame "RBRACKET" {
          }
          frame "RCONTROL" {
          }
          frame "RETURN" {
          }
          frame "R ALT" {
          }
          frame "RSHIFT" {
          }
          frame "RWIN" {
          }
          frame "SCROLL" {
          }
          frame "SEMICOLON" {
          }
          frame "SLASH" {
          }
          frame "SPACE" {
          }
          frame "SUBTRACT" {
          }
          frame "TAB" {
          }
          frame "DIVIDE" {
          }
          frame "DELETE" {
          }
          frame "DECIMAL" {
          }
          frame "COMMA" {
          }
          frame "CAPITAL" {
          }
          frame "BACKSLASH" {
          }
          frame "BACK" {
          }
          frame "ADD" {
          }
          frame "F15" {
          }
          frame "F14" {
          }
          frame "F13" {
          }
          frame "F12" {
          }
          frame "F11" {
          }
          frame "F10" {
          }
          frame "F9" {
          }
          frame "F8" {
          }
          frame "F7" {
          }
          frame "F6" {
          }
          frame "F5" {
          }
          frame "F4" {
          }
          frame "F3" {
          }
          frame "F2" {
          }
          frame "F1" {
          }
          frame "Z" {
          }
          frame "Y" {
          }
          frame "X" {
          }
          frame "W" {
          }
          frame "V" {
          }
          frame "U" {
          }
          frame "T" {
          }
          frame "S" {
          }
          frame "R" {
          }
          frame "Q" {
          }
          frame "P" {
          }
          frame "O" {
          }
          frame "N" {
          }
          frame "M" {
          }
          frame "L" {
          }
          frame "K" {
          }
          frame "J" {
          }
          frame "I" {
          }
          frame "H" {
          }
          frame "G" {
          }
          frame "F" {
          }
          frame "E" {
          }
          frame "D" {
          }
          frame "C" {
          }
          frame "B" {
          }
          frame "A" {
          }
          frame "9" {
          }
          frame "8" {
          }
          frame "7" {
          }
          frame "6" {
          }
          frame "5" {
          }
          frame "4" {
          }
          frame "3" {
          }
          frame "2" {
          }
          frame "1" {
          }
          frame "0" {
          }
        }
        n918 = Bundle(w398, w397, w412, w411, 0.0) -> (w410:cluster{dbl, dbl, dbl, dbl, dbl})  [unwired: 1 in]
        n919 = Bundle("X"=w420, "Y"=w419) -> (w414:cluster{"X":sgl, "Y":sgl})  [unwired: 1 in]
        n920 = Divide(x=20, y=w381) -> (x/y=w384:sgl)
        n921 = local write "Zoom"(w415) -> ()
        n922 = property on="Image Out" class="ImageControl"("Image Center Position"=w414) -> ()  [unwired: 2 in, 2 out]
        n923 = call "IMAQ Convert Rectangle to ROI (Polygon)"("Rectangle"=w410) -> ("ROI Descriptor"=w408:T2)  [unwired: 7 in, 2 out]
        n924 = Bundle("Application Font", w384, w388, w388, w388, w388, w388, TRUE, w386) -> (w390:T11)  [unwired: 1 in]
        n925 = property on="Image Out 2" class="ImageControl"("ROI"=w408) -> ()  [unwired: 2 in, 2 out]
        n926 = Bundle(w386, w390, w386, w386) -> (w389:T12)  [unwired: 1 in]
        n927 = for {
          N: w436 -> [_]
          shift-right: [w701] -> _
          shift-left: w437 -> [w701]
          shift-right: [w699] -> w422
          shift-left: w435 -> [w698]
          tunnel: w423 -> [w697]
          shift-right: [w694] -> _
          shift-left: w391 -> [w696]
          tunnel: w389 -> [w689]
          i -> [w693]
          n928 = Index Array(array=w701, index=w693) -> (element=w710:T13)
          n929 = Unbundle(w710) -> ("Points"=w709:i32[])  [unwired: 2 out]
          n930 = Array To Cluster(array=w709) -> (cluster=w708:T14)
          n931 = Unbundle(w708) -> ("Points[0]"=w688:i32, "Points[1]"=w685:i32, "Points[2]"=w700:i32, "Points[3]"=w706:i32)  [unwired: 5 out]
          n932 = Add(x=w688, y=10) -> (x+y=w686:i32)
          n933 = Subtract(x=w685, y=w706) -> (x-y=w705:i32)
          n934 = Subtract(x=w688, y=w700) -> (x-y=w707:i32)
          n935 = Square(x=w705) -> (x^2=w703:i32)
          n936 = Square(x=w707) -> (x^2=w704:i32)
          n937 = Add(x=w704, y=w703) -> (x+y=w702:i32)
          n938 = Square Root(x=w702) -> (sqrt(x)=w679:dbl)
          n939 = Multiply(x=w679, y=0.5) -> (x*y=w682:dbl)
          n940 = Add(x=w682, y=w685) -> (x+y=w684:dbl)
          n941 = Bundle(w686, w684) -> (w695:cluster{i32, dbl})  [unwired: 1 in]
          n942 = Multiply(x=w679, y=w697) -> (x*y=w692:dbl[])
          n943 = Index Array(array=w692) -> (element=w691:dbl)  [unwired: 1 in]
          n944 = Number To Fractional String(number=w691) -> (F-format string=w690:string)  [unwired: 3 in]
          n945 = call "IMAQ Overlay Text"("BG Color (Transparent)"=u32 0, "Text Color (black)"=u32 16448250, "Font, Size & Style"=w689, "String"=w690, "Origin"=w695, "Image"=w696) -> ("Image Out"=w694:T1)  [unwired: 4 in, 1 out]
          n946 = Build Array (concatenate)(w698, w692) -> (w699:dbl[])
          n947 = local write "Numeric 3"(w679) -> ()
        }
        n948 = Add Array Elements(numeric array=w422) -> (sum=w433:dbl)
        n949 = local write "Distances"(w422) -> ()
        n950 = local write "Total Width"(w433) -> ()
        n951 = local read "Array 8"() -> (w368:dbl[])
        n952 = local read "Array 7"() -> (w369:dbl[])
        n953 = local read "Width"() -> (w364:dbl)
        n954 = local read "New Dielectric"() -> (w376:dbl)
        n955 = local read "Array 2"() -> (w372:dbl[])
        n956 = local read "Manual"() -> (w362:bool)
        n957 = local read "New Length"() -> (w374:dbl)
        n958 = local read "Array"() -> (w373:dbl[])
        n959 = call "sts_calc_subvi.vi"("Array 2"=w368, "Array"=w369) -> ("STS"=w370:dbl)  [unwired: 9 in]
        n960 = local read "New Width"() -> (w377:dbl)
        n961 = local write "New S.T.S."(w370) -> ()
        n962 = call "mob_calc_subvi.vi"("Width"=w377, "Length"=w374, "Dielectric (d)"=w376, "Array 2"=w372, "Array"=w373) -> ("Vt"=w371:dbl, "Mobility"=w375:dbl)  [unwired: 5 in]
        n963 = Not(x=w362) -> (.not. x?=w360:bool)
        n964 = local write "New Vt"(w371) -> ()
        n965 = local write "New Mobility"(w375) -> ()
        n966 = local read "Total Width"() -> (w366:dbl)
        n967 = Equal To 0?(x=w366) -> (x = 0?=w361:bool)
        n968 = And(x=w361, y=w360) -> (x .and. y?=w359:bool)
        n969 = case shown="True" w359 {
          tunnel: w364 -> [_ w439]
          frame False {
          }
          frame True {
            n970 = local write "New Width"(w439) -> ()
          }
        }
        n971 = Or(x=w361, y=w362) -> (x .or. y?=w365:bool)
        n972 = case shown="True" w365 {
          tunnel: w366 -> [w440 _]
          frame False {
            n973 = local write "New Width"(w440) -> ()
          }
          frame True {
          }
        }
      }
    }
  }
  n974 = disable-structure shown="Disabled" {
    frame Disabled {
      n975 = local read "Folder"() -> ()  [unwired: 1 out]
      n976 = local read "Folder"() -> ()  [unwired: 1 out]
      n977 = local read "Folder"() -> ()  [unwired: 1 out]
    }
    frame Enabled {
    }
  }
